vi "STED Control V9.vi"() -> ()   [LabVIEW 2014]
uses:
  Type Defs/Image Acquisition Parameters.ctl
  Laser Controls.ctl
  Detectors.ctl
  Type Defs/P541.ctl
  Type Defs/M227.ctl
  Type Defs/P612.ctl
  Type Defs/M686.ctl
  Type Defs/P841.ctl
  Type Defs/ASI.ctl
  Type Defs/N664_V2.ctl
  Type Defs/STED Graph Controls.ctl
  Type Defs/Display Controls.ctl
  FPGA-7842R-Reference.ctl
  Manual Controls V2.ctl
  Scan Parameters.ctl
  <vilib>/Utility/miscctls.llb/LVPositionTypeDef.ctl
  Controls/StageStates.ctl
  <vilib>/Utility/miscctls.llb/LVRectTypeDef.ctl
  <vilib>/event_ctls.llb/lveventtype.ctl
  <vilib>/Utility/file.llb/Read From Spreadsheet File (DBL).vi
  <vilib>/Utility/file.llb/Write To Spreadsheet File (DBL).vi
panel:
  in  "Laser Controls 2":T1={"Laser On Time (Ticks)"=15, "Laser Delay (Ticks)"=4}
  out "Channel 6":sgl[][](graph)
  out "Channel 5":sgl[][](graph)
  out "Channel 4":sgl[][](graph)
  out "Channel 3":sgl[][](graph)
  out "Channel 2":sgl[][](graph)
  out "Channel 1":sgl[][](graph)
  in  "Display Controls":T2
  in  "Graph Tools":T3={"Zoom Out"=FALSE, "Zoom In"=FALSE, "Reset Zoom"=FALSE, "Pan Tool"=FALSE, "Show Cursor"=FALSE, "Load File"=FALSE, "Fit Tool"=FALSE, "Smooth Tool"=FALSE, "Merge Tool"=FALSE, "Auto Scale"=FALSE, "Apply Color"=FALSE, "Color Map"=enum."Fire"}
  in  "Shutters":T4
  in  "Upper Objective Z - N664":T5={"Up N664"=FALSE, "Down N664"=FALSE, "Step Size (um)"=0.001, "Position (mm)"=0.0, "Home"=FALSE, "Save"=FALSE} {"Step Size (um)" min=0.001}
  in  "Cavity Translation Z - ASI":T6={"Up ASI"=FALSE, "Down ASI"=FALSE, "Step Size (um)"=0.001, "Z (um)"=0.001, "F (um)"=0.001, "Velocity"=0.001} caption="ASI" {"Velocity" min=0.001; "F (um)" min=0.001; "Z (um)" min=-1500.0 max=1500.0; "Step Size (um)" min=0.001}
  in  "Phase Comp Mirror - P841":T7={"Position (µm)"=0.0, "Step Size (µm)"=1.0, "Up P841"=FALSE, "Down P841"=FALSE}
  in  "Sample Stage XY - M686":T8 {"Y" format="%#_4g"; "X" format="%#_4g"}
  in  "Joystick Velocity":string(combo)
  in  "Radio Buttons":enum32{"Radio Selection 1", "Radio Selection 2"}(radio)
  in  "Bottom Objective XY - P612":T9 {"Y" format="%#_4g"; "X" format="%#_4g"}
  in  "Abort AllStage":bool
  in  "Stages":T10={"M227"=TRUE, "N664"=TRUE, "P612"=TRUE, "M686"=FALSE, "P841"=TRUE, "ASI"=FALSE}
  in  "Sample Z Coarse - M227":T11
  in  "Tab Control":T12(tab)
  in  "SLM":bool
  in  "DM":bool
  in  "Timing":bool
  in  "Camera":bool
  in  "Alignment":bool
  in  "Sample Z - P541":T13={"Step Up"=FALSE, "Step Down"=FALSE, "Z Position"=0.0, "Step Size (um)"=1.0, "Home"=FALSE, "Save"=FALSE}
  in  "Detectors":T14={"PMT"=TRUE, "Far Red (685/40 nm)"=FALSE, "Orange (624/40 nm)"=FALSE, "Green (525/50 nm)"=FALSE, "Sum All"=FALSE}
  in  "Laser Controls":T15 {"STED Power (V)" scale=0.0..10.0}
  in  "Save File Path":path=path "C:/isoSTED_Data/Temp/Test_0000.dbl"
  in  "Capture":bool
  in  "Image Acquisition Parameters":T16={"Scan Type"=enum."Beam Scanning", "Scan Mode"=enum."XY", "Fast Axis Frequency (Hz)"=15780.0, "Image Format"=256, "Line Accumulations"=100, "Frames Per Capture"=1, "Frames Accumulations"=1, "Image Dimension (um)"=[15.0, 15.0], "Number of Z Steps"=1, "Z Steps Size (um)"=1.0, "Pixel Size (nm)"=[58.59375, 58.59375]} {"Z Steps Size (um)" min=0.0; "Number of Z Steps" min=1; "Frames Accumulations" min=1; "Frames Per Capture" min=1; "Line Accumulations" min=1; "Image Format" items=["64 x 64"=64, "128 x 128"=128, "256 x 256"=256, "512 x 512"=512, "1024 x 1024"=1024, "2048 x 2048"=2048]}
  in  "Live":bool
  in  "Exit":bool
  # "Sample Stage XY - M686 (0~25 mm)"
  # "XY"
  # "Z"
  # "Length"
  # "Height"
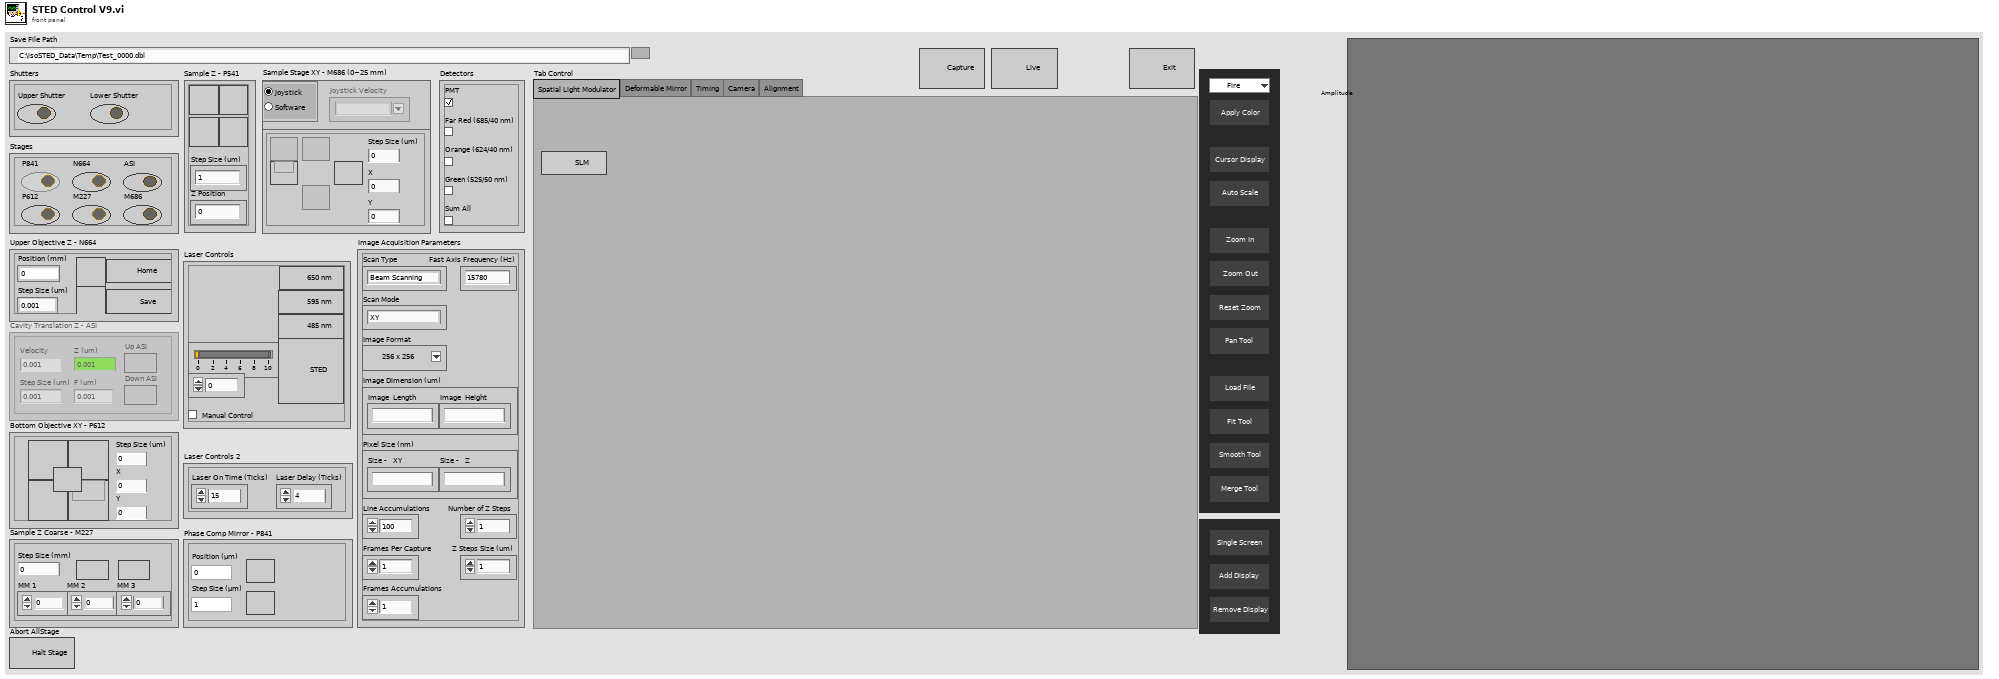
[diagram p1: front panel]
types:
  T1 = cluster{"Laser On Time (Ticks)":i8, "Laser Delay (Ticks)":i8}
  T2 = typedef "Display Controls.ctl" = cluster{"Remove Display":bool, "Add Display":bool, "Single Screen":bool}
  T3 = typedef "STED Graph Controls.ctl" = cluster{"Zoom Out":bool, "Zoom In":bool, "Reset Zoom":bool, "Pan Tool":bool, "Show Cursor":bool, "Load File":bool, "Fit Tool":bool, "Smooth Tool":bool, "Merge Tool":bool, "Auto Scale":bool, "Apply Color":bool, "Color Map":enum16{"System", "Fire", "Gray", "Red", "Green", "Blue", "Cyan", "Magenta", "Yellow", "Red-White", "Green-White", "Blue-White", "Glow"}}
  T4 = cluster{"Upper Shutter":bool, "Lower Shutter":bool}
  T5 = typedef "N664_V2.ctl" = cluster{"Up N664":bool, "Down N664":bool, "Step Size (um)":dbl, "Position (mm)":dbl, "Home":bool, "Save":bool}
  T6 = typedef "ASI.ctl" = cluster{"Up ASI":bool, "Down ASI":bool, "Step Size (um)":dbl, "Z (um)":dbl, "F (um)":dbl, "Velocity":dbl}
  T7 = typedef "P841.ctl" = cluster{"Position (µm)":dbl, "Step Size (µm)":dbl, "Up P841":bool, "Down P841":bool}
  T8 = typedef "M686.ctl" = cluster{"Home Button":bool, "Up Button":bool, "Left Button":bool, "Down Button":bool, "Right Button":bool, "Step Size (um)":dbl, "X":dbl, "Y":dbl}
  T9 = typedef "P612.ctl" = cluster{"Home Button":bool, "Up Button":bool, "Left Button":bool, "Down Button":bool, "Right Button":bool, "Step Size (um)":dbl, "X":dbl, "Y":dbl}
  T10 = cluster{"M227":bool, "N664":bool, "P612":bool, "M686":bool, "P841":bool, "ASI":bool}
  T11 = typedef "M227.ctl" = cluster{"Up M227":bool, "Down M227":bool, "Step Size (mm)":dbl, "MM 1":dbl, "MM 2":dbl, "MM 3":dbl}
  T12 = enum32{"Spatial Light Modulator", "Deformable Mirror", "Timing", "Camera", "Alignment"}
  T13 = typedef "P541.ctl" = cluster{"Step Up":bool, "Step Down":bool, "Z Position":dbl, "Step Size (um)":dbl, "Home":bool, "Save":bool}
  T14 = typedef "Detectors.ctl" = cluster{"PMT":bool, "Far Red (685/40 nm)":bool, "Orange (624/40 nm)":bool, "Green (525/50 nm)":bool, "Sum All":bool}
  T15 = typedef "Laser Controls.ctl" = cluster{"STED Power (V)":dbl, "STED":bool, "650 nm":bool, "590 nm":bool, "485 nm":bool, "Manual Control":bool}
  T16 = typedef "Image Acquisition Parameters.ctl" = cluster{"Scan Type":enum16{"Sample Scanning", "Beam Scanning"}, "Scan Mode":enum16{"XY", "XZ", "YZ", "XYZ"}, "Fast Axis Frequency (Hz)":dbl, "Image Format":u16, "Line Accumulations":u16, "Frames Per Capture":u16, "Frames Accumulations":u16, "Image Dimension (um)":dbl[], "Number of Z Steps":u8, "Z Steps Size (um)":dbl, "Pixel Size (nm)":dbl[]}
  T17 = typedef "Scan Parameters.ctl" = cluster{"Fast_Ax_Amp_V":dbl, "Fast_Ax_Off_V":dbl, "Slow_Ax_Amp_V":dbl, "Slow_Ax_Off_V ":dbl, "Slow_Ax_Max_V_VperS":dbl, "Slow_Ax1_Del25ns":i32, "Slow_Ax2_Del25ns":i32, "Stage_X_Off_V":dbl, "Stage_Y_Off_V":dbl, "Stage_Z_Off_V":dbl, "Galvo1_Off_V":dbl, "Galvo2_Off_V":dbl, "Last_Scan_Mode":enum16{"XY", "XZ", "YZ", "XYZ"}, "Current_Scan_Mode":enum16{"XY", "XZ", "YZ", "XYZ"}, "Fly_Back_Lines":u16, "Linear_Ramp_End":u32, "Z_Step_I16":i16, "Z_Start_I16":i16, "Laser_States _U32":u32, "590_Voltage_I16":i16, "775_AOM_Volt_I16":i16, "Blanking OFF":bool, "Unused_Axis_I16":i16}
  T18 = typedef "Manual Controls V2.ctl" = cluster{"Galvo 1 Position (I16)":i16, "Galvo 2 Position (I16)":i16, "X Axis Voltage (I16)":i16, "Y Axis Voltage (I16)":i16, "Z Axis Voltage (I16)":i16, "Res Mirror Amp (I16)":i16, "Res Mirror Mute":bool, "Upper Shutter":bool, "Lower Shutter":bool}
  T19 = typedef "FPGA-7842R-Reference.ctl" = enum16{"Stage Control", "Laser Control", "Unused Axis I16", "Exit", "Set Res Mirror", "Set Galvo", "Default", "Close FPGA", "Stop Waveforms", "Start Waveforms", "Shutter Control", "Initialize"}
  T20 = enum8{"Enabled", "Disabled", "Disabled and Grayed Out"}
  T21 = typedef "StageStates.ctl" = enum16{"POSITION", "MVR", "MOVE", "HALT", "ONTARGET", "ERROR", "EXIT", "HOME", "ZEROPOS", "NANOPOS", "QUIT", "ANALOG"}
  T22 = typedef "LVRectTypeDef.ctl" = cluster{"Left":i16, "Top":i16, "Right":i16, "Bottom":i16}
  T23 = enum32{"Invalid", "Standard", "Closed", "Hidden", "Minimized", "Maximized"}
  T24 = typedef "lveventtype.ctl" = enum32{"Null", "Timeout", "Annotation Menu Selection", "Annotation Menu Selection?", "App Instance Close", "App Instance Close?", "Autoscale Range Change", "Bookmark Info Change", "Cell Edit", "Cell Edit?", "Cursor Grab", "Cursor Grab?", "Cursor Menu Selection", "Cursor Menu Selection?", "Cursor Move", "Cursor Release", "Data Change", "Direction Change", "Display State Change", "Drag Ended", "Drag Enter", "Drag Leave", "Drag Over", "Drag Source Update", "Drag Starting", "Drag Starting?", "Drop", "Exec State Change", "Key Down", "Key Down?", "Key Repeat", "Key Repeat?", "Key Up", "Listbox Double Click", "Menu Activation?", "Menu Selection (App)", "Menu Selection? (App)", "Menu Selection (User)", "Mouse Down", "Mouse Down?", "Mouse Enter", "Mouse Leave", "Mouse Move", "Mouse Up", "Mouse Wheel", "NI Security User Change (App)", "Pane Size", "Panel Close", "Panel Close?", "Panel Resize", "Plot Attribute Change", "Scale Range Change", "Shortcut Menu Activation?", "Shortcut Menu Selection (App)", "Shortcut Menu Selection? (App)", "Shortcut Menu Selection (User)", "Tree Double Click", "Tree Drag", "Tree Drag?", "Tree Drop", "Tree Drop?", "Tree Item Close", "Tree Item Close?", "Tree Item Open", "Tree Item Open?", "User Event", "Value Change"}
  T25 = typedef "LVPositionTypeDef.ctl" = cluster{"Left":i32, "Top":i32}
  T26 = cluster{"Upper Shutter":bool, "Upper Shutter":bool}
  T27 = cluster{bool, bool, dbl, "Numeric":dbl, "Numeric":dbl, "Numeric":dbl}
  T28 = cluster{"Down_N664":bool, "Down_N664":bool, "Step Size (um)":dbl, "Numeric":dbl, bool, bool}
  T29 = cluster{bool, bool, bool, bool, bool, dbl, "Numeric":dbl, "Numeric":dbl}
  T30 = cluster{"Scan Type":bool, "Scan Mode":bool, "Fast Axis Frequency (Hz)":bool, "Image Format":bool, "Line Accumulations":bool, "Frames Per Capture":bool, "Frames Accumulations":bool, "Image Dimension (um)":bool[], "Number of Z Steps":bool, "Z Steps Size (um)":bool, "Pixel Size (nm)":bool[]}
  T31 = typedef "LVAllMonitorsDisplayTypeDef.ctl" = cluster{"Bounds":cluster{"Left":i16, "Top":i16, "Right":i16, "Bottom":i16}, "Depth":i16}[]
  T32 = cluster{"Bounds":cluster{"Left":i16, "Top":i16, "Right":i16, "Bottom":i16}, "Depth":i16}
  T33 = enum16{"System", "Fire", "Gray", "Red", "Green", "Blue", "Cyan", "Magenta", "Yellow", "Red-White", "Green-White", "Blue-White", "Glow"}
  T34 = typedef "LVPointDoubleTypeDef.ctl" = cluster{"Cursor X":dbl, "Cursor Y":dbl}
  T35 = typedef "LVRangeTypeDef.ctl" = cluster{"Minimum":dbl, "Maximum":dbl, "Increment":dbl, "Minor Increment":dbl, "Start":dbl}
  T36 = typedef "IMAQ Image.ctl" = refnum<image>
  T37 = typedef "Waveform Data.ctl" = cluster{"Waveform Scan Parameters":cluster{"Scanning Mode":u8, "Fast Axis WF Length (Elements)":i32, "Fast Axis Sample Period (Ticks)":u32, "Slow Axis 1 WF Length (Elements)":i32, "Slow Axis 1 Sample Period (Ticks)":u32, "Slow Axis 1 Delay (25 ns) Steps":i32, "Slow Axis 2 WFLength (Elements)":i32, "Slow Axis 2 Sample Period (Ticks)":u32, "Slow Axis 2 Delay (25 ns) Steps":i32}, "Fast Axis Waveform":dbl[], "Slow Axis 1 Waveform":dbl[], "Slow Axis 2 Waveform":dbl[]}
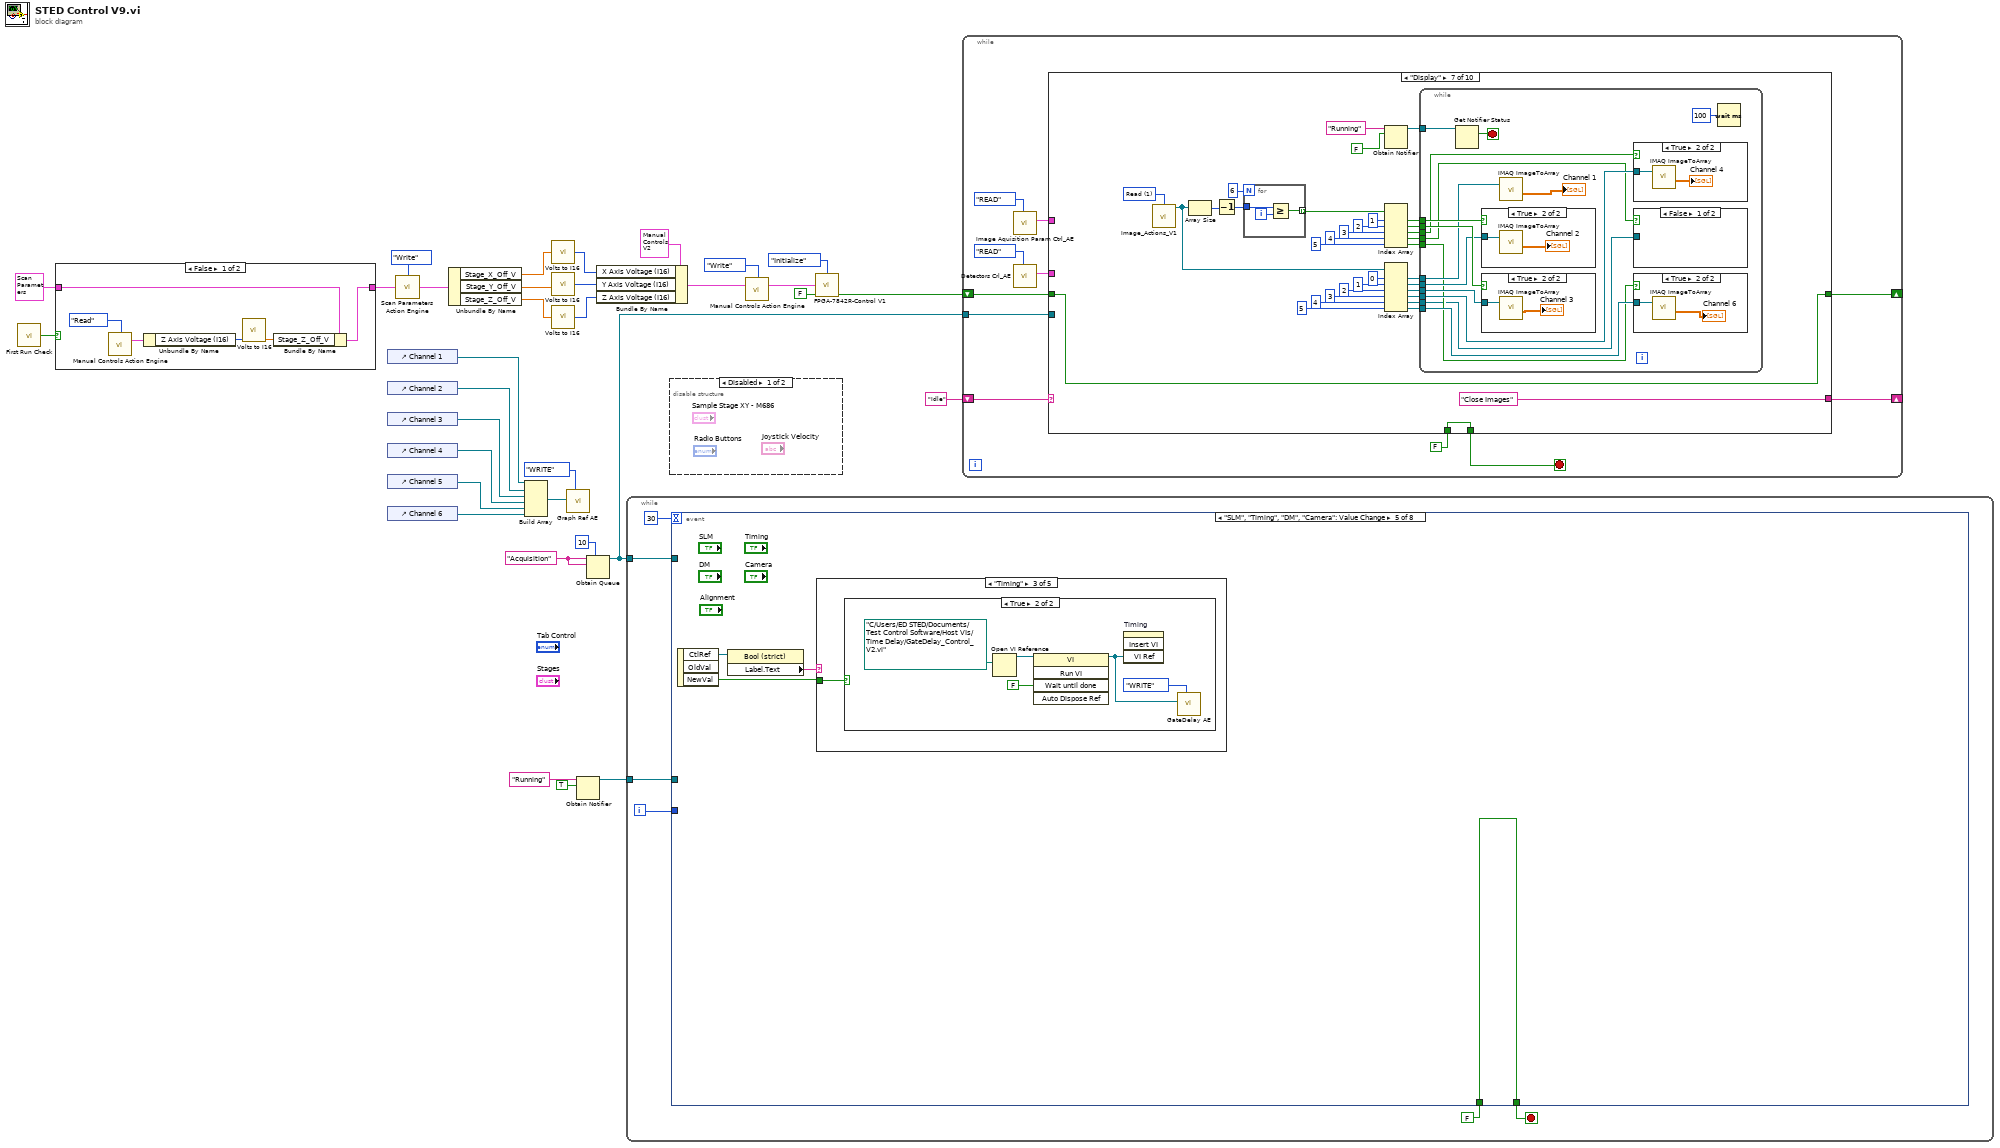
[diagram p0: block diagram]
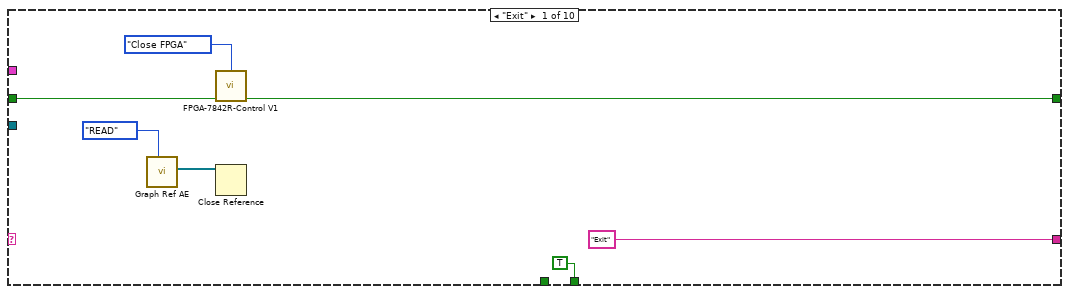
[diagram p4: hidden frame]
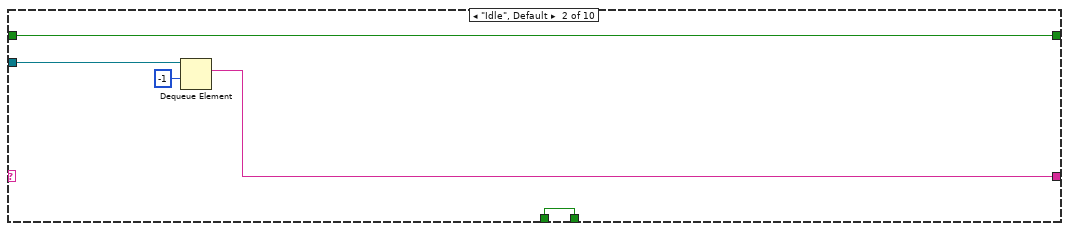
[diagram p5: hidden frame]
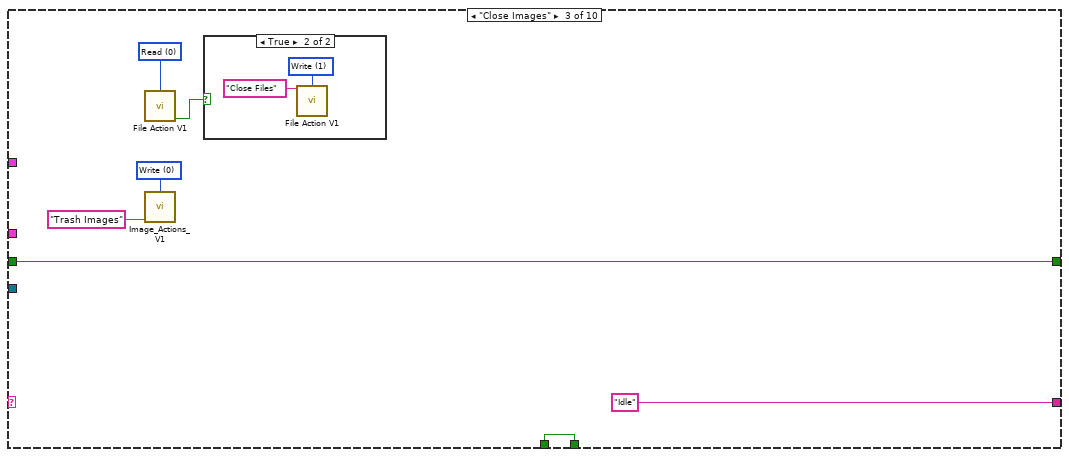
[diagram p6: hidden frame]
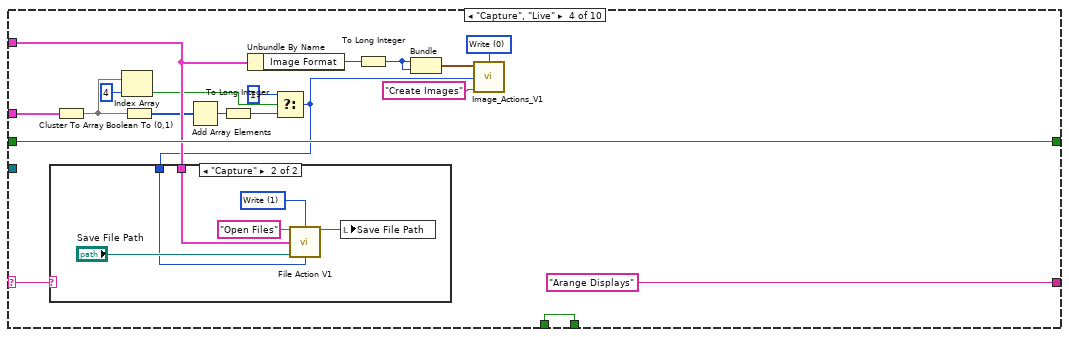
[diagram p8: hidden frame]
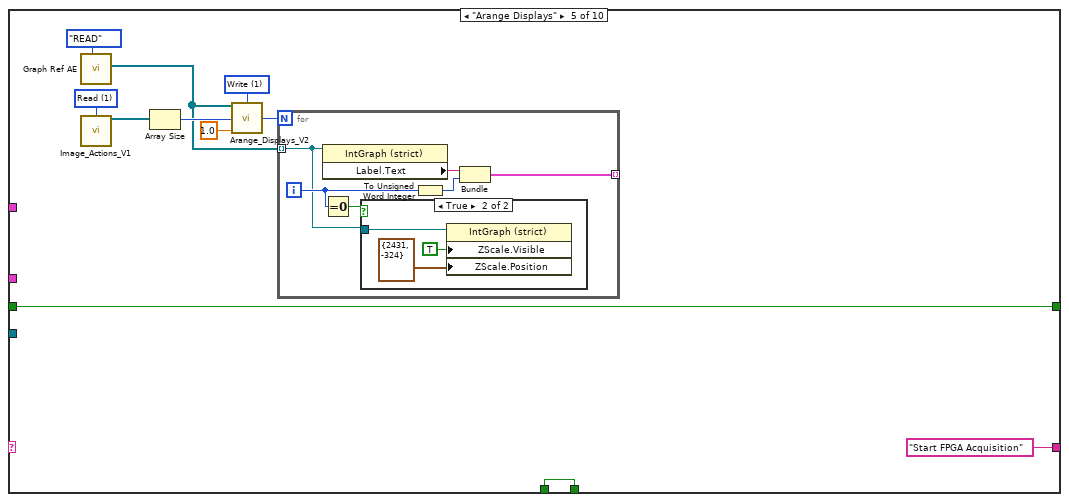
[diagram p10: hidden frame]
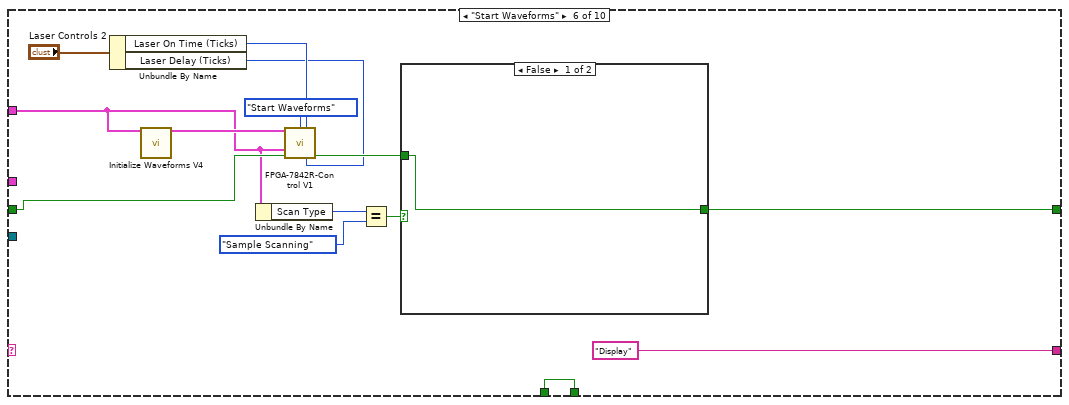
[diagram p12: hidden frame]
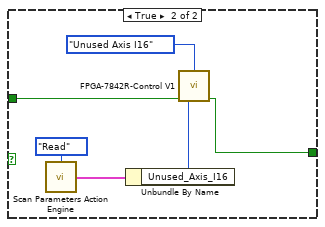
[diagram p13: hidden frame]
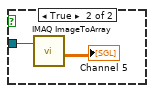
[diagram p15: hidden frame]
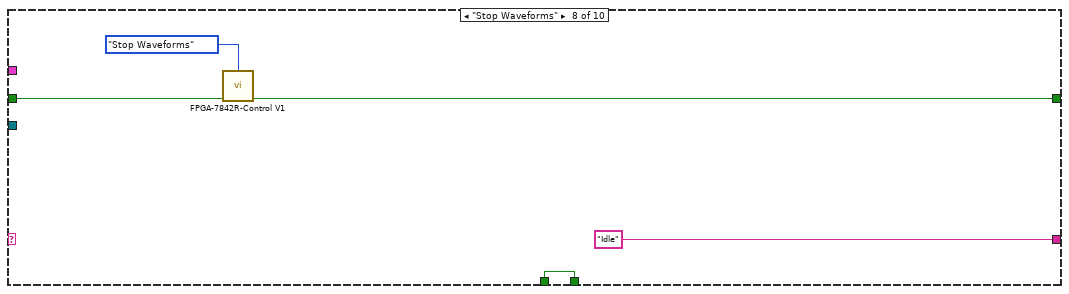
[diagram p19: hidden frame]
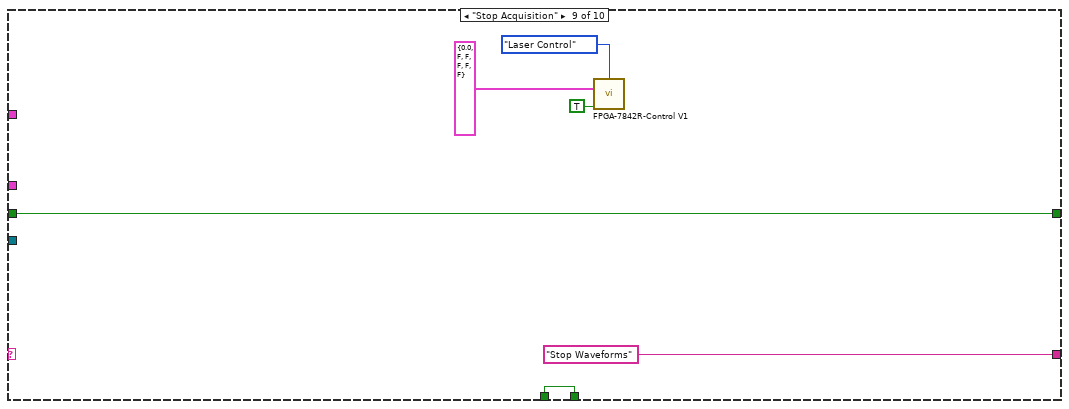
[diagram p20: hidden frame]
diagram:
  w16 = "Acquisition" ("name (unnamed)")
  n1 = call "First Run Check.vi"() -> ("First Run?"=w10:bool)  [unwired: 15 in]
  n2 = case shown="False" w10 {
    tunnel: T17 {"Fast_Ax_Amp_V"=0.0, "Fast_Ax_Off_V"=0.0, "Slow_Ax_Amp_V"=0.0, "Slow_Ax_Off_V "=0.0, "Slow_Ax_Max_V_VperS"=0.0, "Slow_Ax1_Del25ns"=0, "Slow_Ax2_Del25ns"=0, "Stage_X_Off_V"=5.0, "Stage_Y_Off_V"=5.0, "Stage_Z_Off_V"=5.0, "Galvo1_Off_V"=0.0, "Galvo2_Off_V"=0.0, "Last_Scan_Mode"=enum."XY", "Current_Scan_Mode"=enum."XY", "Fly_Back_Lines"=0, "Linear_Ramp_End"=0, "Z_Step_I16"=0, "Z_Start_I16"=0, "Laser_States _U32"=0, "590_Voltage_I16"=0, "775_AOM_Volt_I16"=0, "Blanking OFF"=FALSE, "Unused_Axis_I16"=16384} ("Scan Parameters IN") -> [w39 w40]
    tunnel: [w34 w40] -> w8
    frame False {
      n3 = call "Manual Controls Action Engine.vi"("Action"=enum16{"Read", "Write"}."Read") -> ("Manual Controls Out"=w37:T18)  [unwired: 14 in]
      n4 = Unbundle By Name(w37) -> ("Z Axis Voltage (I16)"=w38:i16)
      n5 = call "Volts to I16.vi"("Volatge (I16)"=w38) -> ("Voltage (V)"=w35:dbl)  [unwired: 13 in, 1 out]
      n6 = Bundle By Name(cluster=w39, "Stage_Z_Off_V"=w35) -> (w34:T17)
    }
    frame True {
    }
  }
  n7 = control-ref of="Channel 1"() -> (w5:refnum<vi>)
  n8 = control-ref of="Channel 2"() -> (w6:refnum<vi>)
  n9 = control-ref of="Channel 3"() -> (w7:refnum<vi>)
  n10 = control-ref of="Channel 4"() -> (w2:refnum<vi>)
  n11 = control-ref of="Channel 5"() -> (w4:refnum<vi>)
  n12 = control-ref of="Channel 6"() -> (w3:refnum<vi>)
  n13 = call "Scan Parameters Action Engine.vi"("Action"=enum16{"Read", "Write"}."Write", "Scan Parameters IN"=w8) -> ("Scan Parameters OUT"=w26:T17)  [unwired: 13 in]
  n14 = Unbundle By Name(w26) -> ("Stage_X_Off_V"=w22:dbl, "Stage_Y_Off_V"=w21:dbl, "Stage_Z_Off_V"=w20:dbl)
  n15 = Build Array(w5, w6, w7, w2, w4, w3) -> (w1:refnum<vi>[])
  n16 = call "Volts to I16.vi"("Voltage (V)"=w22) -> ("I16"=w23:i16)  [unwired: 13 in, 1 out]
  n17 = call "Volts to I16.vi"("Voltage (V)"=w21) -> ("I16"=w24:i16)  [unwired: 13 in, 1 out]
  n18 = call "Volts to I16.vi"("Voltage (V)"=w20) -> ("I16"=w25:i16)  [unwired: 13 in, 1 out]
  n19 = call "Graph Ref AE.vi"("Action"=enum16{"READ", "WRITE"}."WRITE", "Graph Ref In"=w1) -> ()  [unwired: 9 in, 1 out]
  n20 = Obtain Notifier(name (unnamed)="Running", notification data type=TRUE) -> (notifier out=w12:refnum<notifier>)  [unwired: 2 in, 2 out]
  n21 = Obtain Queue(max queue size (-1, unlimited)=10, name (unnamed)=w16, element data type=w16) -> (queue out=w18:refnum<queue>)  [unwired: 2 in, 2 out]
  n22 = Bundle By Name(cluster=T18 {"Galvo 1 Position (I16)"=-280, "Galvo 2 Position (I16)"=0, "X Axis Voltage (I16)"=16384, "Y Axis Voltage (I16)"=16384, "Z Axis Voltage (I16)"=16384, "Res Mirror Amp (I16)"=0, "Res Mirror Mute"=FALSE, "Upper Shutter"=FALSE, "Lower Shutter"=FALSE} ("Manual Controls"), "X Axis Voltage (I16)"=w23, "Y Axis Voltage (I16)"=w24, "Z Axis Voltage (I16)"=w25) -> (w27:T18)
  n23 = while {
    tunnel: w18 -> [w44]
    tunnel: w12 -> [w41]
    i -> [w42]
    stop <- w46 stop-if-true
    n24 = event shown="[4] \"SLM\", \"Timing\", \"DM\", \"Camera\": Value Change" {
      selector: _ -> [_ _ _ _ _ _ _ _]
      dyn-events: _ -> [_ _ _ _ _ _ _ _]
      timeout: 30 -> [_ _ _ _ _ _ _ _]
      tunnel: [w54 w183 w196 w322 w601 w678 w872 w925] -> w46
      tunnel: FALSE -> [w54 w183 w196 w322 w601 w678 w872 _]
      tunnel: w44 -> [w51 w182 _ _ _ _ _ w924]
      tunnel: w42 -> [w49 _ _ _ _ _ _ _]
      tunnel: w41 -> [w47 w175 _ _ _ _ _ w918]
      event Timeout {
        n25 = event-data() -> ()  [unwired: 1 in, 3 out]
        n26 = Equal To 0?(x=w49) -> (x = 0?=w48:bool)
        n27 = Get Notifier Status(notifier=w47) -> (current notification=w53:bool)  [unwired: 1 in, 4 out]
        n28 = case shown="True" w48 {
          frame False {
            w55 = enum16{"WRITE", "READ", "HOME", "SAVE HOME"}."READ" ("Enum")
            n29 = call "Image Aquisition Param Ctrl_AE.vi"("Action"=enum16{"READ", "WRITE"}."READ") -> ("Image Acquisition Parameters Out"=w83:T16)  [unwired: 10 in]
            n30 = call "Detectors Crl_AE.vi"("Action"=enum16{"READ", "WRITE"}."READ") -> ("Detectors Parameters Out"=w84:T14)  [unwired: 10 in]
            n31 = call "LASERs_ Crl_AE.vi"("Action"=enum16{"READ", "WRITE"}."READ") -> ("Detectors Parameters Out"=w85:T15)  [unwired: 10 in]
            n32 = local write "Image Acquisition Parameters"(w83) -> ()
            n33 = local write "Detectors"(w84) -> ()
            n34 = local write "Laser Controls"(w85) -> ()
            n35 = call "Stage_position_ae.vi"("StageID"="M227", "Enum"=w55) -> ("Position Out"=w61:dbl[])  [unwired: 8 in, 1 out]
            n36 = call "Stage_position_ae.vi"("StageID"="P612", "Enum"=w55) -> ("Position Out"=w78:dbl[])  [unwired: 8 in, 1 out]
            n37 = call "Stage_position_ae.vi"("StageID"="P841", "Enum"=w55) -> ("Position Out"=w71:dbl[])  [unwired: 8 in, 1 out]
            n38 = call "Stage_position_ae.vi"("StageID"="N664", "Enum"=w55) -> ("Position Out"=w65:dbl[])  [unwired: 8 in, 1 out]
            n39 = Index Array(array=w65, index=0) -> (element=w64:dbl)
            n40 = Index Array(array=w71, index=0) -> (element=w68:dbl)
            n41 = Index Array(array=w78, index #1=0 ("index"), index #2=1 ("index"), index #3=2 ("index")) -> (element #1=w77:dbl, element #2=w74:dbl, element #3=w72:dbl)
            n42 = Index Array(array=w61, index #1=0 ("index"), index #2=1 ("index"), index #3=2 ("index")) -> (element #1=w58:dbl, element #2=w57:dbl, element #3=w56:dbl)
            n43 = property on="Position (µm)" class="DigNum (strict)"("Value"=w68) -> ()  [unwired: 2 in, 2 out]
            n44 = property on="Position (mm)" class="DigNum (strict)"("Value"=w64) -> ()  [unwired: 2 in, 2 out]
            n45 = property on="X" class="DigNum (strict)"("Value"=w77) -> ()  [unwired: 2 in, 2 out]
            n46 = property on="Y" class="DigNum (strict)"("Value"=w74) -> ()  [unwired: 2 in, 2 out]
            n47 = property on="MM 1" class="DigNum (strict)"("Value"=w58) -> ()  [unwired: 2 in, 2 out]
            n48 = property on="MM 2" class="DigNum (strict)"("Value"=w57) -> ()  [unwired: 2 in, 2 out]
            n49 = property on="Z Position" class="DigNum (strict)"("Value"=w72) -> ()  [unwired: 2 in, 2 out]
            n50 = property on="MM 3" class="DigNum (strict)"("Value"=w56) -> ()  [unwired: 2 in, 2 out]
          }
          frame True {
            w87 = enum16{"WRITE", "READ", "HOME", "SAVE HOME"}."SAVE HOME" ("Enum")
            w99 = FALSE ("Upper Shutter")
            n51 = local read "Image Acquisition Parameters"() -> (w106:T16)
            n52 = local read "Laser Controls"() -> (w104:T15)
            n53 = local read "Detectors"() -> (w103:T14)
            n54 = Bundle("Upper Shutter"=w99, "Upper Shutter"=w99) -> (w100:T26)  [unwired: 1 in]
            n55 = property on="Shutters" class="Clust (strict)"("Value"=w100) -> ()  [unwired: 2 in, 2 out]
            n56 = call "Image Aquisition Param Ctrl_AE.vi"("Action"=enum16{"READ", "WRITE"}."WRITE", "Image Acquisition Parameters In"=w106) -> ()  [unwired: 9 in, 1 out]
            n57 = call "Detectors Crl_AE.vi"("Action"=enum16{"READ", "WRITE"}."WRITE", "Detectors Parameters In"=w103) -> ()  [unwired: 9 in, 1 out]
            n58 = call "LASERs_ Crl_AE.vi"("Action"=enum16{"READ", "WRITE"}."WRITE", "Detectors Parameters In"=w104) -> ()  [unwired: 9 in, 1 out]
            n59 = property on="Stages" class="Clust (strict)"() -> ("Controls[]"=w101:refnum<vi>[])  [unwired: 2 in, 2 out]
            n60 = for {
              tunnel: w101 -> [w111] mode=indexing
              n61 = property class="Ctl"(reference=w111) -> ("Label.Text"=w109:string, "Value"=w113:variant)  [unwired: 1 in, 2 out]
              n62 = Variant To Data(type=TRUE, Variant=w113) -> (data=w110:bool)  [unwired: 1 in, 1 out]
              n63 = call "All_Stages_Aloha.vi"("Aloha"=w110, "Stage ID"=w109) -> ("Position Out"=w108:dbl[])  [unwired: 9 in]
              n64 = case shown="\"N664\"" w109 {
                tunnel: w108 -> [_ w120 w128 w135 w145 w156 w166]
                frame "0", Default {
                }
                frame "M227" {
                  w124 = FALSE
                  n65 = Index Array(array=w120, index #1=0 ("index"), index #2=1 ("index"), index #3=2 ("index")) -> (element #1=w116:dbl, element #2=w115:dbl, element #3=w114:dbl)
                  n66 = Bundle(w124, w124, 0.0, "Numeric"=w116, "Numeric"=w115, "Numeric"=w114) -> (w122:T27)  [unwired: 1 in]
                  n67 = To Variant(anything=w122) -> (Variant=w121:variant)
                  n68 = property on="Sample Z Coarse - M227" class="Clust"("Value"=w121) -> ()  [unwired: 2 in, 2 out]
                }
                frame "N664" {
                  w125 = FALSE
                  w131 = FALSE ("Down_N664")
                  n69 = Index Array(array=w128, index=0) -> (element=w129:dbl)
                  n70 = Bundle("Down_N664"=w131, "Down_N664"=w131, "Step Size (um)"=1.0, "Numeric"=w129, w125, w125) -> (w127:T28)  [unwired: 1 in]
                  n71 = To Variant(anything=w127) -> (Variant=w126:variant)
                  n72 = property on="Upper Objective Z - N664" class="Clust"("Value"=w126) -> ()  [unwired: 2 in, 2 out]
                }
                frame "P612" {
                  w143 = FALSE
                  n73 = Index Array(array=w135, index #1=0, index #2=1, index #3=2 ("index")) -> (element #1=w140:dbl, element #2=w138:dbl, element #3=w133:dbl)
                  n74 = Bundle(w143, w143, w143, w143, w143, 1.0, "Numeric"=w140, "Numeric"=w138) -> (w139:T29)  [unwired: 1 in]
                  n75 = To Variant(anything=w139) -> (Variant=w134:variant)
                  n76 = property on="Bottom Objective XY - P612" class="Clust"("Value"=w134) -> ()  [unwired: 2 in, 2 out]
                  n77 = property on="Z Position" class="DigNum (strict)"("Value"=w133) -> ()  [unwired: 2 in, 2 out]
                }
                frame "M686" {
                  w154 = FALSE
                  n78 = Index Array(array=w145, index #1=0, index #2=1) -> (element #1=w151:dbl, element #2=w146:dbl)
                  n79 = Bundle(w154, w154, w154, w154, w154, 10.0, "Numeric"=w151, "Numeric"=w146) -> (w150:T29)  [unwired: 1 in]
                  n80 = To Variant(anything=w150) -> (Variant=w144:variant)
                  n81 = property on="Joystick Velocity" class="CmbBox"("DisabledEnum"=T20."Disabled and Grayed Out" ("Disabled")) -> ()  [unwired: 2 in, 2 out]
                  n82 = property on="Radio Buttons" class="RadioBtnsControl (strict)"("Value"=enum32{"Radio Selection 1", "Radio Selection 2"}."Radio Selection 2" ("Radio Buttons")) -> ()  [unwired: 2 in, 2 out]
                  n83 = property on="Sample Stage XY - M686" class="Clust"("Value"=w144) -> ()  [unwired: 2 in, 2 out]
                }
                frame "P841" {
                  n84 = Index Array(array=w156, index=0) -> (element=w155:dbl)
                  n85 = property on="Position (µm)" class="DigNum (strict)"("Value"=w155) -> ()  [unwired: 2 in, 2 out]
                }
                frame "ASI" {
                  w162 = FALSE
                  n86 = Add Array Elements(numeric array=w166) -> (sum=w168:dbl)
                  n87 = Index Array(array=w166, index #1=0 ("index"), index #2=1 ("index")) -> (element #1=w161:dbl, element #2=w160:dbl)
                  n88 = Divide(x=w168, y=2000.0) -> ()  [unwired: 1 out]
                  n89 = Bundle By Name(cluster=T6 {"Up ASI"=FALSE, "Down ASI"=FALSE, "Step Size (um)"=0.001, "Z (um)"=0.001, "F (um)"=0.001, "Velocity"=0.001} ("Cavity Translation Z - ASI"), "Up ASI"=w162, "Down ASI"=w162, "Step Size (um)"=1.0, "Z (um)"=w161, "F (um)"=w160, "Velocity"=0.1) -> (w158:T6)
                  n90 = To Variant(anything=w158) -> (Variant=w159:variant)
                  n91 = property on="Cavity Translation Z - ASI" class="Clust"("Value"=w159) -> ()  [unwired: 2 in, 2 out]
                }
              }
            }
            n92 = call-poly <vilib>:"Read From Spreadsheet File.vi"("format (%.3f)"="%.4f", "number of rows (all:-1)"=1, "file path (dialog if empty)"=path "C:/Users/ED STED/Documents/Test Control Software/Host VIs/Stages/Stage Positions/home position.csv") -> ("first row"=w96:dbl[])  [unwired: 4 in, 4 out]
            n93 = Index Array(array=w96, index #1=0 ("index"), index #2=1 ("index")) -> (element #1=w92:dbl, element #2=w93:dbl)
            n94 = Build Array(w92) -> (w91:dbl[])
            n95 = Build Array(w93) -> (w89:dbl[])
            n96 = call "Stage_position_ae.vi"("Position In"=w91, "StageID"="P541", "Enum"=w87) -> ()  [unwired: 7 in, 2 out]
            n97 = call "Stage_position_ae.vi"("Position In"=w89, "StageID"="N664", "Enum"=w87) -> ()  [unwired: 7 in, 2 out]
          }
        }
        n98 = local read "Capture"() -> (w52:bool)
        n99 = And(x=w53, y=w52) -> (x .and. y?=w50:bool)
        n100 = case shown="False" w50 {
          tunnel: w51 -> [_ w173]
          frame False {
          }
          frame True {
            n101 = local write "Capture"(FALSE ("Capture")) -> ()
            n102 = Enqueue Element(queue=w173, element="Stop Acquisition" ("f")) -> ()  [unwired: 2 in, 3 out]
            n103 = property on="Live" class="Bool (strict)"("DisabledEnum"=T20."Enabled" ("Disabled")) -> ()  [unwired: 2 in, 2 out]
          }
        }
      }
      event "Live", "Capture": Value Change {
        n104 = event-data() -> ("CtlRef"=w181:refnum<vi>, "NewVal"=w176:bool)  [unwired: 1 in]
        n105 = Not(x=w176) -> (.not. x?=w179:bool)
        n106 = property class="Bool (strict)"(reference=w181) -> ("Label.Text"=w177:string)  [unwired: 1 in, 2 out]
        n107 = Send Notification(notification=w179, notifier=w175) -> ()  [unwired: 1 in, 2 out]
        n108 = case shown="\"Live\"" w177 {
          tunnel: w176 -> [_ w185 w189]
          frame "False", Default {
          }
          frame "Live" {
            n109 = case shown="True" w185 {
              tunnel: [T20."Enabled" ("Disabled") T20."Disabled and Grayed Out" ("Disabled")] -> w184
              frame False {
              }
              frame True {
              }
            }
            n110 = property on="Capture" class="Bool (strict)"("DisabledEnum"=w184) -> ()  [unwired: 2 in, 2 out]
            n111 = property on="Exit" class="Bool"("DisabledEnum"=w184) -> ()  [unwired: 2 in, 2 out]
          }
          frame "Capture" {
            n112 = case shown="True" w189 {
              tunnel: [T20."Enabled" ("Disabled") T20."Disabled and Grayed Out" ("Disabled")] -> w188
              frame False {
              }
              frame True {
              }
            }
            n113 = property on="Live" class="Bool (strict)"("DisabledEnum"=w188) -> ()  [unwired: 2 in, 2 out]
            n114 = property on="Exit" class="Bool"("DisabledEnum"=w188) -> ()  [unwired: 2 in, 2 out]
          }
        }
        n115 = Select(t=w177, s=w176, f="Stop Acquisition") -> (s? t:f=w178:string)
        n116 = Enqueue Element(queue=w182, element=w178) -> ()  [unwired: 2 in, 3 out]
      }
      event "Shutters": Value Change {
        n117 = event-data() -> ("CtlRef"=w195:refnum<vi>, "NewVal"=w194:variant, "OldVal"=w193:variant)  [unwired: 1 in]
        n118 = property class="Clust"(reference=w195) -> ("Label.Text"=w192:string)  [unwired: 1 in, 2 out]
        n119 = case shown="\"Shutters\"" w192 {
          tunnel: w194 -> [_ w207 _ _ _]
          tunnel: w193 -> [_ w205 _ _ _]
          frame Default {
          }
          frame "Image Acquisition Parameters" {
            n120 = Variant To Data(type="Image Acquisition Parameters", Variant=w207) -> (data=w204:T16)  [unwired: 1 in, 1 out]
            n121 = Variant To Data(type=w204, Variant=w205) -> (data=w203:T16)  [unwired: 1 in, 1 out]
            n122 = Not Equal?(x=w204, y=w203) -> (x != y?=w229:T30)
            n123 = Unbundle By Name(w229) -> ("Image Dimension (um)"=w214:bool[], "Image Format"=w212:bool, "Pixel Size (nm)"=w213:bool[])
            n124 = Or Array Elements(Boolean array=w214) -> (logical OR=w218:bool)
            n125 = Or Array Elements(Boolean array=w213) -> (logical OR=w217:bool)
            n126 = Build Array(w218, w212, w217) -> (w216:bool[])
            n127 = Boolean Array To Number(Boolean array=w216) -> (number=w215:u32)
            n128 = case shown="1, 2" w215 {
              tunnel: w214 -> [_ w251 _]
              tunnel: w204 -> [w239 w244 w259]
              tunnel: [w239 w242 w257] -> w211
              tunnel: w213 -> [_ _ w256]
              tunnel: [w238 w241 w255] -> w210
              tunnel: [w237 w240 w254] -> w208
              frame 0, Default {
                n129 = Unbundle By Name(w239) -> ("Image Dimension (um)"=w238:dbl[], "Scan Mode"=w237:enum16{"XY", "XZ", "YZ", "XYZ"})
              }
              frame 1, 2 {
                # "Image Dimension or Format Change"
                n130 = Unbundle By Name(w244) -> ("Image Dimension (um)"=w250:dbl[], "Image Format"=w248:u16, "Scan Mode"=w240:enum16{"XY", "XZ", "YZ", "XYZ"})
                n131 = for {
                  tunnel: w251 -> [w253] mode=indexing
                  tunnel: w250 -> [w252] mode=indexing
                  tunnel: [w252] -> w249
                  stop <- w253 stop-if-true
                }
                n132 = To Double Precision Float(number=w248) -> (double precision float=w247:dbl)
                n133 = Build Array(w249, w249) -> (w241:dbl[])
                n134 = Divide(x=w241, y=w247) -> (x/y=w246:dbl[])
                n135 = Multiply(x=w246, y=1000.0) -> (x*y=w243:dbl[])
                n136 = Bundle By Name(cluster=w244, "Image Dimension (um)"=w241, "Pixel Size (nm)"=w243) -> (w242:T16)
              }
              frame 4 {
                # "Pixel Size Change"
                n137 = Unbundle By Name(w259) -> ("Pixel Size (nm)"=w265:dbl[], "Image Format"=w263:u16, "Scan Mode"=w254:enum16{"XY", "XZ", "YZ", "XYZ"})
                n138 = for {
                  tunnel: w256 -> [w267] mode=indexing
                  tunnel: w265 -> [w266] mode=indexing
                  tunnel: [w266] -> w264
                  stop <- w267 stop-if-true
                }
                n139 = Build Array(w264, w264) -> (w258:dbl[])
                n140 = To Double Precision Float(number=w263) -> (double precision float=w262:dbl)
                n141 = Multiply(x=w258, y=w262) -> (x*y=w261:dbl[])
                n142 = Multiply(x=w261, y=0.001) -> (x*y=w255:dbl[])
                n143 = Bundle By Name(cluster=w259, "Pixel Size (nm)"=w258, "Image Dimension (um)"=w255) -> (w257:T16)
              }
            }
            n144 = Index Array(array=w210, index=0) -> (element=w234:dbl)
            n145 = Not Equal?(x=enum16{"XY", "XZ", "YZ", "XYZ"}."YZ" ("y"), y=w208) -> (x != y?=w219:bool)
            n146 = call "Res Mirror um to Volts.vi"("Image Size (um)"=w234) -> ("Voltage (V)"=w197:dbl)
            n147 = Select(t=15780.0, s=w219, f=200.0) -> (s? t:f=w222:dbl)
            n148 = In Range and Coerce(upper limit=5.0, x=w197, lower limit=0.0) -> (coerced(x)=w199:dbl)  [unwired: 1 out]
            n149 = call "Scan Parameters Action Engine.vi"("Action"=enum16{"Read", "Write"}."Read") -> ("Scan Parameters OUT"=w200:T17)  [unwired: 14 in]
            n150 = Bundle By Name(cluster=w200, "Fast_Ax_Amp_V"=w199) -> (w198:T17)
            n151 = Bundle By Name(cluster=w211, "Fast Axis Frequency (Hz)"=w222) -> (w221:T16)
            n152 = call "Volts to I16.vi"("Voltage (V)"=w199) -> ("I16"=w233:i16)  [unwired: 13 in, 1 out]
            n153 = call "Scan Parameters Action Engine.vi"("Action"=enum16{"Read", "Write"}."Write", "Scan Parameters IN"=w198) -> ()  [unwired: 13 in, 1 out]
            n154 = call "Manual Controls Action Engine.vi"("Action"=enum16{"Read", "Write"}."Read") -> ("Manual Controls Out"=w227:T18)  [unwired: 14 in]
            n155 = Bundle By Name(cluster=w227, "Res Mirror Amp (I16)"=w233, "Res Mirror Mute"=w219) -> (w225:T18)
            n156 = call "Image Aquisition Param Ctrl_AE.vi"("Action"=enum16{"READ", "WRITE"}."WRITE", "Image Acquisition Parameters In"=w221) -> ()  [unwired: 9 in, 1 out]
            n157 = call "FPGA-7842R-Control V1.vi"("Action"=FPGA-7842R-Reference."Set Res Mirror", "Manual Controls"=w225, "Initialize"=TRUE) -> ()  [unwired: 11 in, 2 out]
            n158 = call "Manual Controls Action Engine.vi"("Action"=enum16{"Read", "Write"}."Write", "Manual Controls In"=w225) -> ()  [unwired: 13 in, 1 out]
          }
          frame "Detectors" {
            n159 = call "Detectors Crl_AE.vi"("Action"=enum16{"READ", "WRITE"}."WRITE", "Detectors Parameters In"="Detectors") -> ()  [unwired: 9 in, 1 out]
          }
          frame "Laser Controls" {
            w282 = FALSE ("element")
            n160 = Unbundle By Name("Laser Controls") -> ("STED"=w288:bool, "650 nm"=w285:bool, "590 nm"=w286:bool, "485 nm"=w287:bool, "STED Power (V)"=w279:dbl, "Manual Control"=w273:bool)
            n161 = local read "Live"() -> (w274:bool)
            n162 = call "LASERs_ Crl_AE.vi"("Action"=enum16{"READ", "WRITE"}."WRITE", "Detectors Parameters In"="Laser Controls") -> ()  [unwired: 9 in, 1 out]
            n163 = Or(x=w274, y=w273) -> (x .or. y?=w272:bool)
            n164 = In Range and Coerce(upper limit=10.0, x=w279, lower limit=0.0) -> (coerced(x)=w276:dbl)  [unwired: 1 out]
            n165 = Build Array(w288, w285, w286, w287, w282, w282, w282, w282) -> (w284:bool[])
            n166 = case shown="True" w272 {
              tunnel: "Laser Controls" -> [_ w294]
              frame False {
              }
              frame True {
                n167 = call "FPGA-7842R-Control V1.vi"("Action"=FPGA-7842R-Reference."Laser Control", "Laser Controls"=w294, "Initialize"=TRUE) -> ()  [unwired: 11 in, 2 out]
              }
            }
            n168 = Boolean Array To Number(Boolean array=w284) -> (number=w283:u32)
            n169 = To Unsigned Byte Integer(number=w283) -> (unsigned 8bit integer=w281:u8)
            n170 = call "U8_To_U32.vi"("U8 IN"=w281) -> ("U32 OUT"=w280:u32)  [unwired: 13 in, 1 out]
            n171 = call "Volts to I16.vi"("Voltage (V)"=w276) -> ("I16"=w275:i16)  [unwired: 13 in, 1 out]
            n172 = call "Scan Parameters Action Engine.vi"("Action"=enum16{"Read", "Write"}."Read") -> ("Scan Parameters OUT"=w291:T17)  [unwired: 14 in]
            n173 = Bundle By Name(cluster=w291, "Laser_States _U32"=w280, "775_AOM_Volt_I16"=w275) -> (w289:T17)
            n174 = call "Scan Parameters Action Engine.vi"("Action"=enum16{"Read", "Write"}."Write", "Scan Parameters IN"=w289) -> ()  [unwired: 13 in, 1 out]
          }
          frame "Shutters" {
            n175 = Unbundle By Name("Shutters") -> ("Upper Shutter"=w306:bool, "Lower Shutter"=w305:bool)
            n176 = Not(x=w306) -> (.not. x?=w297:bool)
            n177 = Not(x=w305) -> (.not. x?=w296:bool)
            n178 = call "Manual Controls Action Engine.vi"("Action"=enum16{"Read", "Write"}."Read") -> ("Manual Controls Out"=w301:T18)  [unwired: 14 in]
            n179 = Bundle By Name(cluster=w301, "Upper Shutter"=w297, "Lower Shutter"=w296) -> (w298:T18)
            n180 = call "Manual Controls Action Engine.vi"("Action"=enum16{"Read", "Write"}."Write", "Manual Controls In"=w298) -> ()  [unwired: 13 in, 1 out]
            n181 = call "FPGA-7842R-Control V1.vi"("Action"=FPGA-7842R-Reference."Shutter Control", "Manual Controls"=w298, "Initialize"=TRUE) -> ()  [unwired: 11 in, 2 out]
          }
        }
      }
      event Value Change {
        # "For P541 - Sample Z - Converting from Step in µm to I16 is as follows. We have (Step µw)*(10 V / 100 µm)*(32768 I16 / 10 V) = (Step µm)*(32768 I16 / 100 µm) = (Step µm)*(327.68 I16/µm)"
        n182 = event-data() -> ("CtlRef"=w320:refnum<vi>, "OldVal"=w318:variant, "NewVal"=w319:variant)  [unwired: 1 in]
        n183 = local write "Abort AllStage"(FALSE ("Abort AllStage")) -> ()
        n184 = property class="Clust"(reference=w320) -> ("Label.Text"=w317:string)  [unwired: 1 in, 2 out]
        n185 = case shown="\"Upper Objective Z - N664\"" w317 {
          tunnel: w319 -> [_ w343 w384 w411 w474 w515 w544]
          tunnel: w318 -> [_ w342 w383 w410 w475 w516 w545]
          tunnel: ["" "N664" "ASI" "P612" "P612" "P841" "M227"] -> w316
          tunnel: [dbl[] [0.0] w334 w376 w399 dbl[] [0.0] w504 w537] -> w315
          tunnel: [bool[] [FALSE] w332 w370 w400 bool[] [FALSE] bool[] [TRUE] w538] -> w314
          tunnel: [enum16{"MOVE", "MVR"}."MVR" ("MOVE/MVR") w331 w373 w402 enum16{"MOVE", "MVR"}."MVR" ("MOVE/MVR") w507 w530] -> w313
          tunnel: [0.0 ("Step Size (um)") 0.5 ("Step Size (um)") w375 0.0 ("Velocity") 0.0 ("Velocity") 10000.0 ("Velocity") 0.0 ("Velocity")] -> w309
          tunnel: [StageStates."MVR" ("Action") w329 w374 w403 StageStates."POSITION" ("Action") w508 w534] -> w307
          frame Default {
          }
          frame "Upper Objective Z - N664" {
            n186 = call "N664_Ctrl_Index.vi"("OldVal"=w342, "NewVal"=w343) -> ("Control Ref OUT"=w341:refnum<vi>, "N664 Out"=w339:T5)  [unwired: 12 in]
            n187 = property class="Ctl"(reference=w341) -> ("Label.Text"=w340:string)  [unwired: 1 in, 2 out]
            n188 = Unbundle By Name(w339) -> ("Step Size (um)"=w338:dbl, "Position (mm)"=w337:dbl)
            n189 = case shown="\"Save\"" w340 {
              tunnel: w338 -> [_ w348 w351 _ _ _]
              tunnel: [0.0 ("Step Size (um)") w347 w351 w356 w358 w363] -> w335
              tunnel: w337 -> [_ _ _ w356 w358 _]
              tunnel: [enum16{"MOVE", "MVR"}."MVR" ("MOVE/MVR") enum16{"MOVE", "MVR"}."MVR" ("MOVE/MVR") enum16{"MOVE", "MVR"}."MVR" ("MOVE/MVR") enum16{"MOVE", "MVR"}."MOVE" ("MOVE/MVR") enum16{"MOVE", "MVR"}."MOVE" ("MOVE/MVR") enum16{"MOVE", "MVR"}."MOVE" ("MOVE/MVR")] -> w331
              tunnel: [StageStates."MVR" ("Action") StageStates."MVR" ("Action") StageStates."MVR" ("Action") StageStates."MOVE" ("Action") StageStates."MOVE" ("Action") StageStates."MOVE" ("Action")] -> w329
              frame Default {
              }
              frame "Up N664" {
                n190 = Negate(x=w348) -> (-x=w347:dbl)
              }
              frame "Down N664" {
              }
              frame "Position (mm)" {
              }
              frame "Save" {
                n191 = Build Array(w358) -> (w357:dbl[])
                n192 = call "Stage_position_ae.vi"("Position In"=w357, "StageID"="N664", "Enum"=enum16{"WRITE", "READ", "HOME", "SAVE HOME"}."SAVE HOME") -> ()  [unwired: 7 in, 2 out]
              }
              frame "Home" {
                n193 = call "Stage_position_ae.vi"("StageID"="N664", "Enum"=enum16{"WRITE", "READ", "HOME", "SAVE HOME"}."HOME") -> ("Position Out"=w365:dbl[])  [unwired: 8 in, 1 out]
                n194 = Index Array(array=w365, index=0) -> (element=w363:dbl)
              }
            }
            n195 = Build Array(w335) -> (w334:dbl[])
            n196 = Build Array(TRUE) -> (w332:bool[])
          }
          frame "Cavity Translation Z - ASI" {
            n197 = call "ASI_Ctrl_Index.vi"("NewVal"=w384, "OldVal"=w383) -> ("ASI out"=w380:T6, "Control Ref OUT"=w382:refnum<vi>)  [unwired: 8 in]
            n198 = property class="Ctl"(reference=w382) -> ("Label.Text"=w381:string)  [unwired: 1 in, 2 out]
            n199 = Unbundle By Name(w380) -> ("Step Size (um)"=w379:dbl, "Z (um)"=w378:dbl, "Velocity"=w375:dbl)
            n200 = case shown="\"Z (um)\"" w381 {
              tunnel: w379 -> [_ w390 w393 _]
              tunnel: w378 -> [_ _ _ w397]
              tunnel: [0.0 ("Z (um)") w390 w394 w397] -> w377
              tunnel: [StageStates."MVR" ("Action") StageStates."MVR" ("Action") StageStates."MVR" ("Action") StageStates."MOVE" ("Action")] -> w374
              tunnel: [enum16{"MOVE", "MVR"}."MVR" ("MOVE/MVR") enum16{"MOVE", "MVR"}."MVR" ("MOVE/MVR") enum16{"MOVE", "MVR"}."MVR" ("MOVE/MVR") enum16{"MOVE", "MVR"}."MOVE" ("MOVE/MVR")] -> w373
              frame Default {
              }
              frame "Up ASI" {
              }
              frame "Down ASI" {
                n201 = Negate(x=w393) -> (-x=w394:dbl)
              }
              frame "Z (um)" {
              }
            }
            n202 = Build Array(w377) -> (w376:dbl[])
            n203 = Build Array(TRUE) -> (w370:bool[])
          }
          frame "Bottom Objective XY - P612" {
            n204 = call "P612_Ctrl_Index.vi"("OldVal"=w410, "NewVal"=w411) -> ("Control out"=w409:refnum<vi>, "P612 out"=w407:T9)  [unwired: 12 in]
            n205 = property class="Ctl"(reference=w409) -> ("Label.Text"=w408:string)  [unwired: 1 in, 2 out]
            n206 = Unbundle By Name(w407) -> ("Step Size (um)"=w406:dbl, "X"=w405:dbl, "Y"=w404:dbl)
            n207 = case shown="\"Up Button\"" w408 {
              tunnel: w406 -> [_ _ w422 w429 w433 w440 _]
              tunnel: w405 -> [_ _ _ _ _ _ w447]
              tunnel: w404 -> [_ _ _ _ _ _ w446]
              tunnel: [StageStates."MVR" ("Action") StageStates."HOME" ("Action") StageStates."MVR" ("Action") StageStates."MVR" ("Action") StageStates."MVR" ("Action") StageStates."MVR" ("Action") StageStates."MOVE" ("Action")] -> w403
              tunnel: [enum16{"MOVE", "MVR"}."MVR" ("MOVE/MVR") enum16{"MOVE", "MVR"}."MVR" ("MOVE/MVR") enum16{"MOVE", "MVR"}."MVR" ("MOVE/MVR") enum16{"MOVE", "MVR"}."MVR" ("MOVE/MVR") enum16{"MOVE", "MVR"}."MVR" ("MOVE/MVR") enum16{"MOVE", "MVR"}."MVR" ("MOVE/MVR") enum16{"MOVE", "MVR"}."MOVE" ("MOVE/MVR")] -> w402
              tunnel: [bool[] [FALSE] bool[] [TRUE, TRUE] bool[] [TRUE, FALSE] bool[] [TRUE, FALSE] bool[] [FALSE, TRUE] bool[] [FALSE, TRUE] bool[] [TRUE, TRUE]] -> w400
              tunnel: [dbl[] [0.0] dbl[] [0.0, 0.0] w421 w428 w435 w442 w448] -> w399
              frame Default {
              }
              frame "Home Button" {
              }
              frame "Up Button" {
                n208 = Build Array(w422, 0.0 ("element")) -> (w421:dbl[])
              }
              frame "Down Button" {
                n209 = Negate(x=w429) -> (-x=w426:dbl)
                n210 = Build Array(w426, 0.0 ("element")) -> (w428:dbl[])
              }
              frame "Left Button" {
                n211 = Build Array(0.0 ("element"), w433) -> (w435:dbl[])
              }
              frame "Right Button" {
                n212 = Negate(x=w440) -> (-x=w439:dbl)
                n213 = Build Array(0.0 ("element"), w439) -> (w442:dbl[])
              }
              frame "X", "Y" {
                n214 = Build Array(w447, w446) -> (w448:dbl[])
              }
            }
          }
          frame "Sample Z - P541" {
            w453 = 327.68 ("y")
            n215 = call "P541_Ctrl_Index.vi"("OldVal"=w475, "NewVal"=w474) -> ("Control out"=w473:refnum<vi>, "P541 Out"=w472:T13)  [unwired: 12 in]
            n216 = Unbundle By Name(w472) -> ("Z Position"=w452:dbl, "Step Size (um)"=w471:dbl)
            n217 = property class="Ctl"(reference=w473) -> ("Label.Text"=w470:string)  [unwired: 1 in, 2 out]
            n218 = call "Manual Controls Action Engine.vi"("Action"=enum16{"Read", "Write"}."Read") -> ("Manual Controls Out"=w461:T18)  [unwired: 14 in]
            n219 = Unbundle By Name(w461) -> ("Z Axis Voltage (I16)"=w464:i16)
            n220 = Multiply(x=w452, y=w453) -> (x*y=w467:dbl)
            n221 = Multiply(x=w471, y=w453) -> (x*y=w469:dbl)
            n222 = Round To Nearest(number=w467) -> (nearest integer value=w456:dbl)
            n223 = Round To Nearest(number=w469) -> (nearest integer value=w455:dbl)
            n224 = To Word Integer(number=w456) -> (16bit integer=w466:i16)
            n225 = To Word Integer(number=w455) -> (16bit integer=w468:i16)
            n226 = case shown="\"Home\"" w470 {
              tunnel: w468 -> [_ w482 w486 _ _ _]
              tunnel: w466 -> [_ _ _ w488 _ _]
              tunnel: w464 -> [w481 w484 w487 _ w493 _]
              tunnel: [w481 w483 w485 w488 w493 w499] -> w460
              tunnel: w453 -> [_ _ _ _ _ w498]
              tunnel: w452 -> [_ _ _ _ w492 _]
              frame Default {
              }
              frame "Step Down" {
                n227 = Subtract(x=w484, y=w482) -> (x-y=w483:i16)
              }
              frame "Step Up" {
                n228 = Add(x=w487, y=w486) -> (x+y=w485:i16)
              }
              frame "Z Position" {
              }
              frame "Save" {
                n229 = Build Array(w492) -> (w491:dbl[])
                n230 = call "Stage_position_ae.vi"("Position In"=w491, "StageID"="P541", "Enum"=enum16{"WRITE", "READ", "HOME", "SAVE HOME"}."SAVE HOME") -> ()  [unwired: 7 in, 2 out]
              }
              frame "Home" {
                n231 = call "Stage_position_ae.vi"("StageID"="P541", "Enum"=enum16{"WRITE", "READ", "HOME", "SAVE HOME"}."HOME") -> ("Position Out"=w496:dbl[])  [unwired: 8 in, 1 out]
                n232 = Index Array(array=w496, index=0) -> (element=w494:dbl)
                n233 = Multiply(x=w494, y=w498) -> (x*y=w500:dbl)
                n234 = Round To Nearest(number=w500) -> (nearest integer value=w501:dbl)
                n235 = To Word Integer(number=w501) -> (16bit integer=w499:i16)
              }
            }
            n236 = Bundle By Name(cluster=w461, "Z Axis Voltage (I16)"=w460) -> (w463:T18)
            n237 = call "Manual Controls Action Engine.vi"("Action"=enum16{"Read", "Write"}."Write", "Manual Controls In"=w463) -> ("Manual Controls Out"=w457:T18)  [unwired: 13 in]
            n238 = call "FPGA-7842R-Control V1.vi"("Action"=FPGA-7842R-Reference."Stage Control", "Manual Controls"=w457, "Initialize"=TRUE) -> ()  [unwired: 11 in, 2 out]
          }
          frame "Phase Comp Mirror - P841" {
            n239 = call "P841_Ctrl_Index.vi"("OldVal"=w516, "NewVal"=w515) -> ("Control out"=w513:refnum<vi>, "P841 Out"=w511:T7)  [unwired: 12 in]
            n240 = property class="Ctl"(reference=w513) -> ("Label.Text"=w512:string)  [unwired: 1 in, 2 out]
            n241 = Unbundle By Name(w511) -> ("Position (µm)"=w510:dbl, "Step Size (µm)"=w509:dbl)
            n242 = case shown="\"Down P841\"" w512 {
              tunnel: w510 -> [_ _ _ w529]
              tunnel: w509 -> [_ w522 w526 _]
              tunnel: [0.0 ("Position (µm)") w522 w525 w529] -> w505
              tunnel: [StageStates."MVR" ("Action") StageStates."MVR" ("Action") StageStates."MVR" ("Action") StageStates."MOVE" ("Action")] -> w508
              tunnel: [enum16{"MOVE", "MVR"}."MVR" ("MOVE/MVR") enum16{"MOVE", "MVR"}."MVR" ("MOVE/MVR") enum16{"MOVE", "MVR"}."MVR" ("MOVE/MVR") enum16{"MOVE", "MVR"}."MOVE" ("MOVE/MVR")] -> w507
              frame Default {
              }
              frame "Up P841" {
              }
              frame "Down P841" {
                n243 = Negate(x=w526) -> (-x=w525:dbl)
              }
              frame "Position (µm)" {
              }
            }
            n244 = Build Array(w505) -> (w504:dbl[])
          }
          frame "Sample Z Coarse - M227" {
            n245 = call "M227_Ctrl_Index.vi"("OldVal"=w545, "NewVal"=w544) -> ("Control Ref OUT"=w543:refnum<vi>, "M227 Out"=w541:T11)  [unwired: 12 in]
            n246 = property class="Ctl"(reference=w543) -> ("Label.Text"=w542:string)  [unwired: 1 in, 2 out]
            n247 = Unbundle By Name(w541) -> ("Step Size (mm)"=w540:dbl, "MM 1"=w533:dbl, "MM 2"=w532:dbl, "MM 3"=w531:dbl)
            n248 = case shown="Default" w542 {
              tunnel: w540 -> [_ _ _ _ w564 w569]
              tunnel: [bool[] [FALSE, FALSE, FALSE] bool[] [TRUE, TRUE, TRUE] bool[] [TRUE, TRUE, TRUE] bool[] [TRUE, TRUE, TRUE] bool[] [TRUE, TRUE, TRUE] bool[] [TRUE, TRUE, TRUE]] -> w538
              tunnel: [0.0 ("Step Size (mm)") w551 w555 w559 w564 w568] -> w535
              tunnel: [StageStates."POSITION" ("Action") StageStates."MOVE" ("Action") StageStates."MOVE" ("Action") StageStates."MOVE" ("Action") StageStates."MVR" ("Action") StageStates."MVR" ("Action")] -> w534
              tunnel: w533 -> [_ w551 _ _ _ _]
              tunnel: w532 -> [_ _ w555 _ _ _]
              tunnel: w531 -> [_ _ _ w559 _ _]
              tunnel: [enum16{"MOVE", "MVR"}."MVR" ("MOVE/MVR") enum16{"MOVE", "MVR"}."MOVE" ("MOVE/MVR") enum16{"MOVE", "MVR"}."MOVE" ("MOVE/MVR") enum16{"MOVE", "MVR"}."MOVE" ("MOVE/MVR") enum16{"MOVE", "MVR"}."MVR" ("MOVE/MVR") enum16{"MOVE", "MVR"}."MVR" ("MOVE/MVR")] -> w530
              frame Default {
              }
              frame "MM 1" {
              }
              frame "MM 2" {
              }
              frame "MM 3" {
              }
              frame "Up M227" {
              }
              frame "Down M227" {
                n249 = Negate(x=w569) -> (-x=w568:dbl)
              }
            }
            n250 = Build Array(w535, w535, w535) -> (w537:dbl[])
          }
        }
        n251 = case shown="\"Cavity Translation Z - ASI\"" w317 {
          frame Default {
          }
          frame "Upper Objective Z - N664" {
            n252 = while {
              i -> [w576]
              stop <- w572 stop-if-true
              n253 = call "Stage_position_ae.vi"("StageID"="N664", "Enum"=enum16{"WRITE", "READ", "HOME", "SAVE HOME"}."READ") -> ("Status Out"=w573:bool, "Position Out"=w583:dbl[])  [unwired: 8 in]
              n254 = Greater?(x=w576, y=200) -> (0:w575:bool)
              n255 = And(x=w573, y=w575) -> (x .and. y?=w572:bool)
              n256 = Wait (ms)(milliseconds to wait=u32 1) -> ()  [unwired: 1 out]
              n257 = Index Array(array=w583, index=0) -> (element=w582:dbl)
              n258 = Select(t=u32 16777215, s=w572, f=u32 6618880) -> (s? t:f=w577:u32)
              n259 = property on="Position (mm)" class="DigNum (strict)"("Value"=w582, "NumText.BG Color"=w577) -> ()  [unwired: 2 in, 2 out]
            }
          }
          frame "Cavity Translation Z - ASI" {
            n260 = while {
              shift-right: [w590] -> _
              shift-left: TRUE ("Status Out") -> [w595]
              stop <- w594 stop-if-true
              n261 = call "Stage_position_ae.vi"("StageID"="ASI", "Enum"=enum16{"WRITE", "READ", "HOME", "SAVE HOME"}."READ") -> ("Status Out"=w590:bool, "Position Out"=w598:dbl[])  [unwired: 8 in]
              n262 = Greater?(x=w590, y=w595) -> (0:w594:bool)
              n263 = Wait (ms)(milliseconds to wait=u32 1) -> ()  [unwired: 1 out]
              n264 = Index Array(array=w598, index=0) -> (element=w588:dbl)
              n265 = Divide(x=w588, y=10.0) -> (x/y=w589:dbl)
              n266 = Select(t=u32 16777215, s=w590, f=u32 6618880) -> (s? t:f=w591:u32)
              n267 = property on="Z (um)" class="DigNum (strict)"("Value"=w589, "NumText.BG Color"=w591) -> ()  [unwired: 2 in, 2 out]
            }
          }
        }
        n268 = control-ref of="Abort AllStage"() -> (w308:refnum<vi>)
        n269 = call "AllStage_Limits_Array.vi"("Step(um)/Position(units)"=w315, "Axis"=w314, "Stage ID"=w316, "MOVE/MVR"=w313) -> ("Positions"=w311:dbl[], "Boolean Array"=w310:bool[], "Stage ID"=w312:string)  [unwired: 5 in]
        n270 = call "AE_AllStages_Action V2.vi"("Velocity"=w309, "Abort"=w308, "Positions"=w311, "Axis"=w310, "Stage ID"=w312, "Action"=w307) -> ()  [unwired: 3 in, 3 out]
      }
      event "SLM", "Timing", "DM", "Camera": Value Change {
        n271 = event-data() -> ("CtlRef"=w603:refnum<vi>, "NewVal"=w600:bool)  [unwired: 1 in, 1 out]
        n272 = property class="Bool (strict)"(reference=w603) -> ("Label.Text"=w602:string)  [unwired: 1 in, 2 out]
        n273 = case shown="\"Timing\"" w602 {
          tunnel: w600 -> [w604 w618 w632 w646 w659]
          frame "SLM", Default {
            n274 = case shown="True" w604 {
              frame False {
                n275 = To Variant(anything=TRUE) -> (Variant=w610:variant)
                n276 = call "SLM AE.vi"("Action"=enum16{"READ", "WRITE"}."READ") -> ("SLM Ref Out"=w611:refnum<vi>)  [unwired: 10 in]
                n277 = invoke class="VI" method="Ctrl Val.Set"(reference=w611, "Control Name"="Exit", "Value"=w610) -> (reference out=w607:refnum<vi>, error out=w606:errorcluster)  [unwired: 2 in, 3 out]
                n278 = invoke on="Hamamatsu LCOS" class="SubPnl" method="Remove VI"(error in=w606) -> (error out=w605:errorcluster)  [unwired: 2 in, 2 out]
                n279 = Close Reference(reference=w607, error in (no error)=w605) -> ()  [unwired: 1 out]
              }
              frame True {
                n280 = Open VI Reference(vi path=path "C:/Users/ED STED/Documents/Test Control Software/Host VIs/SLM_V2/SLM Control.vi") -> (vi reference=w616:refnum<vi>)  [unwired: 5 in, 1 out]
                n281 = invoke class="VI" method="Run VI"(reference=w616, "Wait until done"=FALSE ("Wait Until Done")) -> (reference out=w613:refnum<vi>)  [unwired: 3 in, 4 out]
                n282 = invoke on="Hamamatsu LCOS" class="SubPanel" method="Insert VI"("VI Ref"=w613) -> ()  [unwired: 3 in, 4 out]
                n283 = call "SLM AE.vi"("Action"=enum16{"READ", "WRITE"}."WRITE", "SLM Ref In"=w613) -> ()  [unwired: 9 in, 1 out]
              }
            }
          }
          frame "DM" {
            n284 = case shown="False" w618 {
              frame False {
                n285 = call "DM_Ref_AE.vi"("Action"=enum16{"READ", "WRITE"}."READ") -> ("DM Ref Out"=w625:refnum<vi>)  [unwired: 10 in]
                n286 = To Variant(anything=TRUE) -> (Variant=w624:variant)
                n287 = invoke class="VI" method="Ctrl Val.Set"(reference=w625, "Control Name"="Exit", "Value"=w624) -> (reference out=w621:refnum<vi>, error out=w620:errorcluster)  [unwired: 2 in, 3 out]
                n288 = invoke on="BM Multi" class="SubPnl" method="Remove VI"(error in=w620) -> (error out=w619:errorcluster)  [unwired: 2 in, 2 out]
                n289 = Close Reference(reference=w621, error in (no error)=w619) -> ()  [unwired: 1 out]
              }
              frame True {
                n290 = Open VI Reference(vi path=path "C:/Users/ED STED/Documents/Test Control Software/Host VIs/DM_Dual_V2/Dual_DM_Control_Main_V3.vi") -> (vi reference=w630:refnum<vi>)  [unwired: 5 in, 1 out]
                n291 = invoke class="VI" method="Run VI"(reference=w630, "Wait until done"=FALSE ("Wait Until Done")) -> (reference out=w627:refnum<vi>)  [unwired: 3 in, 4 out]
                n292 = invoke on="BM Multi" class="SubPanel" method="Insert VI"("VI Ref"=w627) -> ()  [unwired: 3 in, 4 out]
                n293 = call "DM_Ref_AE.vi"("Action"=enum16{"READ", "WRITE"}."WRITE", "DM Ref In"=w627) -> ()  [unwired: 9 in, 1 out]
              }
            }
          }
          frame "Timing" {
            n294 = case shown="True" w632 {
              frame False {
                n295 = To Variant(anything=TRUE) -> (Variant=w637:variant)
                n296 = call "GateDelay AE.vi"("Action"=enum16{"READ", "WRITE"}."READ") -> ("Gate Delay Ref Out"=w638:refnum<vi>)  [unwired: 10 in]
                n297 = invoke class="VI" method="Ctrl Val.Set"(reference=w638, "Control Name"="Exit", "Value"=w637) -> (reference out=w633:refnum<vi>, error out=w634:errorcluster)  [unwired: 2 in, 3 out]
                n298 = invoke on="Timing" class="SubPnl" method="Remove VI"(error in=w634) -> (error out=w640:errorcluster)  [unwired: 2 in, 2 out]
                n299 = Close Reference(reference=w633, error in (no error)=w640) -> ()  [unwired: 1 out]
              }
              frame True {
                n300 = Open VI Reference(vi path=path "C:/Users/ED STED/Documents/Test Control Software/Host VIs/Time Delay/GateDelay_Control_V2.vi") -> (vi reference=w643:refnum<vi>)  [unwired: 5 in, 1 out]
                n301 = invoke class="VI" method="Run VI"(reference=w643, "Wait until done"=FALSE ("Wait Until Done")) -> (reference out=w642:refnum<vi>)  [unwired: 3 in, 4 out]
                n302 = invoke on="Timing" class="SubPanel" method="Insert VI"("VI Ref"=w642) -> ()  [unwired: 3 in, 4 out]
                n303 = call "GateDelay AE.vi"("Action"=enum16{"READ", "WRITE"}."WRITE", "Gate Delay Ref In"=w642) -> ()  [unwired: 9 in, 1 out]
              }
            }
          }
          frame "Camera" {
            n304 = case shown="True" w646 {
              frame False {
                n305 = To Variant(anything=TRUE) -> (Variant=w647:variant)
                n306 = call "Camera_Ref_HX.vi"("Action"=enum16{"READ", "WRITE"}."READ") -> ("Alignment Ref Out"=w651:refnum<vi>)  [unwired: 10 in]
                n307 = invoke class="VI" method="Ctrl Val.Set"(reference=w651, "Control Name"="Exit", "Value"=w647) -> (reference out=w650:refnum<vi>)  [unwired: 2 in, 4 out]
                n308 = invoke on="uc480" class="SubPnl" method="Remove VI"() -> (error out=w652:errorcluster)  [unwired: 3 in, 2 out]
                n309 = Close Reference(reference=w650, error in (no error)=w652) -> ()  [unwired: 1 out]
              }
              frame True {
                n310 = Open VI Reference(vi path=path "C:/Users/ED STED/Documents/Test Control Software/Host VIs/Camera/uEye_Control_V1.vi") -> (vi reference=w656:refnum<vi>)  [unwired: 5 in, 1 out]
                n311 = invoke class="VI" method="Run VI"(reference=w656, "Wait until done"=FALSE ("Wait Until Done")) -> (reference out=w655:refnum<vi>)  [unwired: 3 in, 4 out]
                n312 = invoke on="uc480" class="SubPnl" method="Insert VI"("VI Ref"=w655) -> ()  [unwired: 3 in, 4 out]
                n313 = call "Camera_Ref_HX.vi"("Action"=enum16{"READ", "WRITE"}."WRITE", "Alignment Ref In"=w655) -> ()  [unwired: 9 in, 1 out]
              }
            }
          }
          frame "Alignment" {
            n314 = case shown="True" w659 {
              frame False {
                n315 = To Variant(anything=TRUE) -> (Variant=w660:variant)
                n316 = call "FocusLock_Ref_HX.vi"("Action"=enum16{"READ", "WRITE"}."READ") -> ("Camera Ref Out"=w664:refnum<vi>)  [unwired: 10 in]
                n317 = invoke class="VI" method="Ctrl Val.Set"(reference=w664, "Control Name"="Exit", "Value"=w660) -> (reference out=w663:refnum<vi>)  [unwired: 2 in, 4 out]
                n318 = invoke on="uc480" class="SubPnl" method="Remove VI"() -> (error out=w665:errorcluster)  [unwired: 3 in, 2 out]
                n319 = Close Reference(reference=w663, error in (no error)=w665) -> ()  [unwired: 1 out]
              }
              frame True {
                n320 = Open VI Reference(vi path=path "C:/Users/ED STED/Documents/Test Control Software/Host VIs/AutoAlign/AutoAlign_SWITCH.vi") -> (vi reference=w669:refnum<vi>)  [unwired: 5 in, 1 out]
                n321 = invoke class="VI" method="Run VI"(reference=w669, "Wait until done"=FALSE ("Wait Until Done")) -> (reference out=w668:refnum<vi>)  [unwired: 3 in, 4 out]
                n322 = invoke on="uc480" class="SubPnl" method="Insert VI"("VI Ref"=w668) -> ()  [unwired: 3 in, 4 out]
                n323 = call "FocusLock_Ref_HX.vi"("Action"=enum16{"READ", "WRITE"}."WRITE", "Camera Ref In"=w668) -> ()  [unwired: 9 in, 1 out]
              }
            }
          }
        }
      }
      event Value Change {
        n324 = event-data() -> ("CtlRef"=w677:refnum<vi>, "OldVal"=w675:variant, "NewVal"=w674:variant)  [unwired: 1 in]
        n325 = property class="Clust"(reference=w677) -> ("Label.Text"=w676:string)  [unwired: 1 in, 2 out]
        n326 = call "Graph Ref AE.vi"("Action"=enum16{"READ", "WRITE"}."READ") -> ("Graph Ref Out"=w672:refnum<vi>[])  [unwired: 10 in]
        n327 = case shown="\"Graph Tools\"" w676 {
          tunnel: w675 -> [_ w684 w740]
          tunnel: w674 -> [_ w685 w739]
          tunnel: w672 -> [_ w679 w732]
          frame Default {
          }
          frame "Display Controls" {
            n328 = call "Display_Controls_Ctrl_Index.vi"("OldVal"=w684, "NewVal"=w685) -> ("Control Ref OUT"=w683:refnum<vi>, "Display Controls Out"=w681:T2)  [unwired: 12 in]
            n329 = property class="Ctl"(reference=w683) -> ("Label.Text"=w682:string)  [unwired: 1 in, 2 out]
            n330 = Unbundle By Name(w681) -> ("Single Screen"=w680:bool)
            n331 = case shown="\"Single Screen\", Default" w682 {
              tunnel: w680 -> [w693 _ _]
              tunnel: w679 -> [_ w718 w725]
              frame "Single Screen", Default {
                n332 = property class="App"() -> ("Disp.AllMonitors"=w692:T31)  [unwired: 2 in, 2 out]
                n333 = Index Array(array=w692, index #1=2 ("index"), index #2=0 ("index")) -> (element #1=w689:T32, element #2=w688:T32)
                n334 = control-ref of="This VI"() -> (w687:refnum<vi>)
                n335 = case shown="False" w693 {
                  tunnel: w689 -> [w697 _]
                  tunnel: w688 -> [w696 w708]
                  tunnel: w687 -> [w695 w706]
                  tunnel: T22 {"Left"=0, "Top"=0, "Right"=0, "Bottom"=0} ("Front Panel Window:Window Bounds") -> [w694 w707]
                  frame False {
                    w702 = i16 0
                    n336 = Unbundle By Name(w696) -> ("Bounds.Left"=w699:i16, "Bounds.Bottom"=w700:i16, "Bounds.Top"=w701:i16)
                    n337 = Unbundle By Name(w697) -> ("Bounds.Right"=w698:i16)
                    n338 = Subtract(x=w698, y=w699) -> (x-y=w703:i16)
                    n339 = Subtract(x=w700, y=w701) -> (x-y=w704:i16)
                    n340 = Bundle By Name(cluster=w694, "Left"=w702, "Top"=w702, "Right"=w703, "Bottom"=w704) -> (w705:T22)
                    n341 = property class="VI"(reference=w695, "Front Panel.WinBounds"=w705) -> ()  [unwired: 1 in, 2 out]
                  }
                  frame True {
                    w711 = i16 0
                    n342 = Unbundle By Name(w708) -> ("Bounds.Right"=w714:i16, "Bounds.Bottom"=w713:i16, "Bounds.Top"=w712:i16)
                    n343 = Subtract(x=w713, y=w712) -> (x-y=w710:i16)
                    n344 = Bundle By Name(cluster=w707, "Left"=w711, "Top"=w711, "Right"=w714, "Bottom"=w710) -> (w709:T22)
                    n345 = property class="VI"(reference=w706, "Front Panel.WinBounds"=w709) -> (reference out=w716:refnum<vi>)  [unwired: 1 in, 1 out]
                    n346 = property class="VI"(reference=w716, "FP.State"=T23."Maximized" ("Front Panel Window:State")) -> ()  [unwired: 1 in, 2 out]
                  }
                }
              }
              frame "Add Display" {
                w719 = u16 0 items=["Read", "Write"] ("Action")
                w723 = u16 1 items=["Read", "Write"] ("Action")
                n347 = property on="Add Display" class="Bool (strict)"("Value"=FALSE) -> ()  [unwired: 2 in, 2 out]
                n348 = call "Arange_Displays_V2.vi"("Action"=w719) -> ("Number of Channels OUT"=w720:i32)  [unwired: 14 in]
                n349 = Increment(x=w720) -> (x+1=w722:i32)
                n350 = call "Arange_Displays_V2.vi"("Display References"=w718, "Action"=w723, "Number of Channels"=w722, "Aspect Ratio (h/w)"=1.0) -> ()  [unwired: 11 in, 1 out]
              }
              frame "Remove Display" {
                w726 = u16 0 items=["Read", "Write"] ("Action")
                w730 = u16 1 items=["Read", "Write"] ("Action")
                n351 = call "Arange_Displays_V2.vi"("Action"=w726) -> ("Number of Channels OUT"=w727:i32)  [unwired: 14 in]
                n352 = Decrement(x=w727) -> (x-1=w729:i32)
                n353 = call "Arange_Displays_V2.vi"("Display References"=w725, "Action"=w730, "Number of Channels"=w729, "Aspect Ratio (h/w)"=1.0) -> ()  [unwired: 11 in, 1 out]
                n354 = property on="Remove Display" class="Bool (strict)"("Value"=FALSE) -> ()  [unwired: 2 in, 2 out]
              }
            }
          }
          frame "Graph Tools" {
            n355 = call "Graph_Controls_Ctrl_Index.vi"("OldVal"=w740, "NewVal"=w739) -> ("Control Ref OUT"=w738:refnum<vi>, "Graph Tools Out"=w737:T3)  [unwired: 12 in]
            n356 = property class="Ctl"(reference=w738) -> (reference out=w734:refnum<vi>, "Label.Text"=w733:string)  [unwired: 1 in, 1 out]
            n357 = Unbundle By Name(w737) -> ("Show Cursor"=w736:bool, "Auto Scale"=w735:bool, "Color Map"=w731:T33)
            n358 = case shown="\"Apply Color\"" w733 {
              selector: w733 -> [_ _ _ w809 _ _ _ _]
              tunnel: w736 -> [_ w778 _ _ _ _ _ _]
              tunnel: w735 -> [_ _ w798 _ _ _ _ _]
              tunnel: w732 -> [w749 w777 w799 w802 w839 _ w851 w859]
              tunnel: w734 -> [_ _ _ _ _ _ _ _]
              tunnel: w733 -> [_ _ _ w804 _ _ _ _]
              tunnel: w731 -> [w752 _ _ _ _ _ _ _]
              frame "Apply Color" {
                n359 = control-ref of="This VI"() -> (w751:refnum<vi>)
                n360 = call "GetDisplayClick.vi"("Display REFs In"=w749, "Calling VI REF"=w751) -> ("Display Index"=w750:i32)  [unwired: 13 in]
                n361 = Index Array(array=w749, index=w750) -> (element=w748:refnum<vi>)
                n362 = property class="IntGraph (strict)"(reference=w748) -> (reference out=w744:refnum<vi>, error out=w741:errorcluster, "ZScale.Maximum"=w747:dbl)  [unwired: 1 in]
                n363 = case shown="\"Gray\"" w752 {
                  tunnel: [cluster{dbl, u32}[] [{0.0, 0}, {85.0, 16711680}, {108.0, 16729344}, {127.0, 16744192}, {132.0, 16747520}, {140.0, 16753920}, {157.0, 16766720}, {170.0, 16776960}, {245.0, 16777184}, {250.0, 16777200}, {255.0, 16777215}] ("Z Scale.Marker Values[]") cluster{dbl, u32}[] [{0.0, 0}, {255.0, 16777215}] ("Z Scale.Marker Values[]") cluster{dbl, u32}[] [{0.0, 0}, {255.0, 16711680}] ("Z Scale.Marker Values[]") cluster{dbl, u32}[] [{0.0, 0}, {255.0, 65280}] ("Z Scale.Marker Values[]") cluster{dbl, u32}[] [{0.0, 0}, {255.0, 255}] ("Z Scale.Marker Values[]") cluster{dbl, u32}[] [{0.0, 0}, {255.0, 65535}] ("Z Scale.Marker Values[]") cluster{dbl, u32}[] [{0.0, 0}, {255.0, 16711935}] ("Z Scale.Marker Values[]") cluster{dbl, u32}[] [{0.0, 0}, {255.0, 16776960}] ("Z Scale.Marker Values[]") cluster{dbl, u32}[] [{0.0, 0}, {170.0, 16711680}, {245.0, 16777184}, {250.0, 16777200}, {255.0, 16448250}] ("Z Scale.Marker Values[]") cluster{dbl, u32}[] [{0.0, 0}, {170.0, 65280}, {245.0, 16777184}, {250.0, 16777200}, {255.0, 16448250}] ("Z Scale.Marker Values[]") cluster{dbl, u32}[] [{0.0, 0}, {170.0, 255}, {245.0, 16777184}, {250.0, 16777200}, {255.0, 16448250}] ("Z Scale.Marker Values[]") cluster{dbl, u32}[] [{0.0, 0}, {1.0, 131072}, {2.0, 196608}, {3.0, 327680}, {4.0, 458752}, {5.0, 589824}, {6.0, 720896}, {7.0, 851971}, {8.0, 983043}, {9.0, 1114115}, {10.0, 1245187}, {11.0, 1376259}, {12.0, 1507331}, {13.0, 1638403}, {14.0, 1769475}, {15.0, 1769479}, {16.0, 2031623}, {17.0, 2162695}, {18.0, 2293767}, {19.0, 2424839}, {20.0, 2555911}, {21.0, 2686983}, {22.0, 2818055}, {23.0, 2949127}, {24.0, 3080203}, {25.0, 3211275}, {26.0, 3342347}, {27.0, 3473419}, {28.0, 3604491}, {29.0, 3735563}, {30.0, 3866635}, {31.0, 3867403}, {32.0, 4129547}, {33.0, 4260619}, {34.0, 4391691}, {35.0, 4522763}, {36.0, 4653839}, {37.0, 4784911}, {38.0, 4915983}, {39.0, 5178127}, {40.0, 5309199}, {41.0, 5440271}, {42.0, 5571343}, {43.0, 5702415}, {44.0, 5703439}, {45.0, 5965583}, {46.0, 6096655}, {47.0, 6227727}, {48.0, 6358799}, {49.0, 6489871}, {50.0, 6620943}, {51.0, 6752015}, {52.0, 6883087}, {53.0, 7015183}, {54.0, 7146255}, {55.0, 7277327}, {56.0, 7408399}, {57.0, 7539471}, {58.0, 7670543}, {59.0, 7801615}, {60.0, 8063759}, {61.0, 8194831}, {62.0, 8326927}, {63.0, 8457999}, {64.0, 8589075}, {65.0, 8720147}, {66.0, 8851219}, {67.0, 8982291}, {68.0, 9113363}, {69.0, 9114387}, {70.0, 9376531}, {71.0, 9507603}, {72.0, 9638675}, {73.0, 9769747}, {74.0, 9901843}, {75.0, 10032915}, {76.0, 10163987}, {77.0, 10229523}, {78.0, 10295059}, {79.0, 10427155}, {80.0, 10558227}, {81.0, 10689299}, {82.0, 10820371}, {83.0, 10886931}, {84.0, 10952467}, {85.0, 11083539}, {86.0, 11214611}, {87.0, 11215635}, {88.0, 11477779}, {89.0, 11543315}, {90.0, 11608851}, {91.0, 11740947}, {92.0, 11806483}, {93.0, 11872019}, {94.0, 12004115}, {95.0, 12135187}, {96.0, 12266259}, {97.0, 12267283}, {98.0, 12398355}, {99.0, 12529427}, {100.0, 12530451}, {101.0, 12595987}, {102.0, 12530451}, {103.0, 12793619}, {104.0, 12794131}, {105.0, 12794643}, {106.0, 13056787}, {107.0, 13057299}, {108.0, 13057811}, {109.0, 13188883}, {110.0, 13320979}, {111.0, 13386515}, {112.0, 13452563}, {113.0, 13584147}, {114.0, 13584659}, {115.0, 13585171}, {116.0, 13585683}, {117.0, 13717267}, {118.0, 13848339}, {119.0, 13849363}, {120.0, 13849875}, {121.0, 13850387}, {122.0, 13981459}, {123.0, 14113555}, {124.0, 14114067}, {125.0, 14114579}, {126.0, 14115091}, {127.0, 14246675}, {128.0, 14377747}, {129.0, 14378771}, {130.0, 14379283}, {131.0, 14379539}, {132.0, 14379795}, {133.0, 14380819}, {134.0, 14511891}, {135.0, 14643987}, {136.0, 14644503}, {137.0, 14645015}, {138.0, 14645527}, {139.0, 14646039}, {140.0, 14646551}, {141.0, 14778135}, {142.0, 14909207}, {143.0, 14910231}, {144.0, 14910747}, {145.0, 14911259}, {146.0, 14911771}, {147.0, 14912283}, {148.0, 14912797}, {149.0, 15044383}, {150.0, 15175455}, {151.0, 15175967}, {152.0, 15176479}, {153.0, 15176991}, {154.0, 15177507}, {155.0, 15178019}, {156.0, 15178531}, {157.0, 15310115}, {158.0, 15441701}, {159.0, 15441959}, {160.0, 15442215}, {161.0, 15442727}, {162.0, 15443243}, {163.0, 15443755}, {164.0, 15444269}, {165.0, 15444783}, {166.0, 15444783}, {167.0, 15576367}, {168.0, 15707953}, {169.0, 15708467}, {170.0, 15708979}, {171.0, 15708981}, {172.0, 15708983}, {173.0, 15710011}, {174.0, 15710523}, {175.0, 15711037}, {176.0, 15711039}, {177.0, 15711553}, {178.0, 15843139}, {179.0, 15974213}, {180.0, 15974215}, {181.0, 15974217}, {182.0, 15974219}, {183.0, 15975755}, {184.0, 15976271}, {185.0, 15976785}, {186.0, 15977299}, {187.0, 15977301}, {188.0, 15977815}, {189.0, 15978327}, {190.0, 15978331}, {191.0, 16109917}, {192.0, 16241503}, {193.0, 16241505}, {194.0, 16242019}, {195.0, 16242535}, {196.0, 16242537}, {197.0, 16242539}, {198.0, 16243563}, {199.0, 16243567}, {200.0, 16244081}, {201.0, 16244595}, {202.0, 16244599}, {203.0, 16244601}, {204.0, 16244603}, {205.0, 16245627}, {206.0, 16245631}, {207.0, 16245633}, {208.0, 16246147}, {209.0, 16246663}, {210.0, 16377735}, {211.0, 16508811}, {212.0, 16508815}, {213.0, 16509839}, {214.0, 16509843}, {215.0, 16509845}, {216.0, 16509847}, {217.0, 16510361}, {218.0, 16510875}, {219.0, 16510879}, {220.0, 16510881}, {221.0, 16510883}, {222.0, 16511399}, {223.0, 16511911}, {224.0, 16511915}, {225.0, 16511917}, {226.0, 16511919}, {227.0, 16511923}, {228.0, 16512437}, {229.0, 16512951}, {230.0, 16512955}, {231.0, 16512957}, {232.0, 16512959}, {233.0, 16512961}, {234.0, 16512963}, {235.0, 16512967}, {236.0, 16513481}, {237.0, 16513995}, {238.0, 16513999}, {239.0, 16514001}, {240.0, 16514003}, {241.0, 16514005}, {242.0, 16514007}, {243.0, 16514011}, {244.0, 16514013}, {245.0, 16514015}, {246.0, 16514019}, {247.0, 16514021}, {248.0, 16514023}, {249.0, 16514027}, {250.0, 16514029}, {251.0, 16514031}, {252.0, 16514035}, {253.0, 16514037}, {254.0, 16514039}, {255.0, 16514043}] ("Z Scale.Marker Values[]")] -> w743
                  tunnel: w747 -> [w753 w755 w757 w759 w761 w763 w765 w767 w769 w771 w773 w776]
                  tunnel: [w753 w755 w757 w759 w761 w763 w765 w767 w769 w771 w773 w776] -> w745
                  frame "Fire", Default {
                    # "Fire"
                  }
                  frame "Gray" {
                    # "Grayscale"
                  }
                  frame "Red" {
                    # "Red"
                  }
                  frame "Green" {
                    # "Green"
                  }
                  frame "Blue" {
                    # "Blue"
                  }
                  frame "Cyan" {
                    # "Cyan"
                  }
                  frame "Magenta" {
                    # "Magenta"
                  }
                  frame "Yellow" {
                    # "Yellow"
                  }
                  frame "Red-White" {
                    # "Red-White"
                  }
                  frame "Green-White" {
                    # "Green-White"
                  }
                  frame "Blue-White" {
                    # "Blue-White"
                  }
                  frame "Glow" {
                  }
                }
                n364 = property on="Apply Color" class="Bool (strict)"(error in=w741, "Value"=FALSE) -> ()  [unwired: 1 in, 2 out]
                n365 = property class="IntGraph (strict)"(reference=w744, "ZScale.MarkerVals[]"=w743, "ZScale.High Color"=u32 255, "ZScale.Maximum"=w745) -> ()  [unwired: 1 in, 2 out]
              }
              frame "Show Cursor", Default {
                w781 = 2.0 ("y")
                n366 = Index Array(array=w777, index=0) -> (element=w789:refnum<vi>)
                n367 = property class="IntGraph (strict)"(reference=w789) -> ("Value"=w788:sgl[][])  [unwired: 1 in, 2 out]
                n368 = Array Size(array=w788) -> (size(s)=w787:i32[])
                n369 = To Double Precision Float(number=w787) -> (double precision float=w784:dbl[])
                n370 = Index Array(array=w784, index #1=0 ("index"), index #2=1 ("index")) -> (element #1=w783:dbl, element #2=w782:dbl)
                n371 = Divide(x=w783, y=w781) -> (x/y=w780:dbl)
                n372 = Divide(x=w782, y=w781) -> (x/y=w779:dbl)
                n373 = for {
                  tunnel: w777 -> [w791] mode=indexing
                  tunnel: w780 -> [w793]
                  tunnel: w779 -> [w792]
                  tunnel: w778 -> [w794]
                  n374 = property class="IntGraph (strict)"(reference=w791, "Cursor.Visible"=w794, "Cursor.Cursor X"=w793, "Cursor.Cursor Y"=w792) -> ()  [unwired: 1 in, 2 out]
                }
              }
              frame "Auto Scale" {
                n375 = Select(t=u8 2 ("Z Scale.Scale Fit"), s=w798, f=u8 0) -> (s? t:f=w795:u8)
                n376 = for {
                  tunnel: w799 -> [w801] mode=indexing
                  tunnel: w795 -> [w800]
                  n377 = property class="IntGraph (strict)"(reference=w801, "ZScale.ScaleFit"=w800) -> ()  [unwired: 1 in, 2 out]
                }
              }
              frame "Pan Tool", "Reset Zoom", "Zoom In", "Zoom Out" {
                n378 = case shown="\"Reset Zoom\"" w809 {
                  tunnel: [0 ("Palette:Active Tool") 6 ("Palette:Active Tool") 7 ("Palette:Active Tool") 1 ("Palette:Active Tool") 0 ("Palette:Active Tool")] -> w803
                  tunnel: w802 -> [_ _ _ _ w821]
                  frame Default {
                  }
                  frame "Zoom In" {
                  }
                  frame "Zoom Out" {
                  }
                  frame "Pan Tool" {
                  }
                  frame "Reset Zoom" {
                    n379 = property on="Reset Zoom" class="Bool (strict)"("Value"=FALSE) -> ()  [unwired: 2 in, 2 out]
                    n380 = for {
                      tunnel: w821 -> [w826] mode=indexing
                      tunnel: 5 ("Palette:Active Tool") -> [w825]
                      n381 = property class="IntGraph (strict)"(reference=w826, "ActPaletteTool"=w825) -> ()  [unwired: 1 in, 2 out]
                    }
                  }
                }
                n382 = control-ref of="Zoom In"() -> (w805:refnum<vi>)
                n383 = control-ref of="Zoom Out"() -> (w807:refnum<vi>)
                n384 = control-ref of="Pan Tool"() -> (w806:refnum<vi>)
                n385 = Build Array(w805, w807, w806) -> (w808:refnum<vi>[])
                n386 = for {
                  tunnel: w808 -> [w814] mode=indexing
                  tunnel: w804 -> [w812]
                  n387 = property class="Bool (strict)"(reference=w814) -> (reference out=w813:refnum<vi>, "Label.Text"=w811:string)  [unwired: 1 in, 1 out]
                  n388 = Equal?(x=w811, y=w812) -> (x = y?=w810:bool)
                  n389 = property class="Bool (strict)"(reference=w813, "Value"=w810) -> ()  [unwired: 1 in, 2 out]
                }
                n390 = for {
                  tunnel: w802 -> [w816] mode=indexing
                  tunnel: w803 -> [w815]
                  n391 = property class="IntGraph (strict)"(reference=w816, "ActPaletteTool"=w815) -> ()  [unwired: 1 in, 2 out]
                }
              }
              frame "Load File" {
                w836 = u16 1 items=["Get Image", "Load and Read File"] ("Action")
                n392 = control-ref of="This VI"() -> (w838:refnum<vi>)
                n393 = property on="Load File" class="Bool (strict)"("Value"=FALSE) -> ()  [unwired: 2 in, 2 out]
                n394 = call "GetDisplayClick.vi"("Display REFs In"=w839, "Calling VI REF"=w838) -> ("Display Index"=w827:i32)  [unwired: 13 in]
                n395 = call "OpenDBL.vi"("Action"=w836) -> ("Image"=w835:sgl[], "Dimensions (Z, Y, X, t)"=w834:i32[])  [unwired: 11 in, 2 out]
                n396 = Index Array(array=w834, index #1=1 ("index"), index #2=2 ("index")) -> (element #1=w831:i32, element #2=w830:i32)
                n397 = Reverse 1D Array(array=w835) -> (reversed array=w829:sgl[])
                n398 = Reshape Array(w829, w831, w830) -> (w828:sgl[][])
                n399 = Index Array(array=w839, index=w827) -> (element=w837:refnum<vi>)
                n400 = property class="IntGraph (strict)"(reference=w837, "Value"=w828) -> ()  [unwired: 1 in, 2 out]
              }
              frame "Fit Tool" {
                n401 = disable-structure shown="Disabled" {
                  frame Disabled {
                    n402 = vi-ref "QuickProfile_V4.vi"() -> (w843:refnum<vi>)
                    n403 = call "Image Aquisition Param Ctrl_AE.vi"("Action"=enum16{"READ", "WRITE"}."READ") -> ()  [unwired: 10 in, 1 out]
                    n404 = property class="VI Interface Type 0"(reference=w843) -> ("Path"=w846:path)  [unwired: 1 in, 2 out]
                    n405 = Unbundle By Name() -> ("Pixel Size (nm)"=w842:dbl[])  [unwired: 1 in]
                    n406 = Index Array(array=w842, index=0) -> (element=w849:dbl)
                    n407 = Open VI Reference(type specifier VI Refnum (for type only)=w843, vi path=w846, options=128) -> (vi reference=w844:refnum<vi>)  [unwired: 3 in, 1 out]
                    n408 = call-by-ref "Start Asynchronous Call"(reference=w844, "Pixel Size (nm)"=w849) -> (reference out=w847:refnum<vi>)  [unwired: 16 in, 1 out]
                    n409 = Close Reference(reference=w847) -> ()  [unwired: 1 in, 1 out]
                  }
                  frame Enabled {
                  }
                }
              }
              frame "Smooth Tool" {
                n410 = vi-ref "SmoothTool.vi"() -> (w854:refnum<vi>)
                n411 = property on="Smooth Tool" class="Bool (strict)"("Value"=FALSE) -> ()  [unwired: 2 in, 2 out]
                n412 = property class="VI Interface Type 1"(reference=w854) -> ("Path"=w856:path)  [unwired: 1 in, 2 out]
                n413 = control-ref of="This VI"() -> (w852:refnum<vi>)
                n414 = Open VI Reference(type specifier VI Refnum (for type only)=w854, vi path=w856, options=128) -> (vi reference=w855:refnum<vi>)  [unwired: 3 in, 1 out]
                n415 = call-by-ref "Start Asynchronous Call"(reference=w855, "Calling VI REF"=w852, "Display REFs In"=w851) -> (reference out=w853:refnum<vi>)  [unwired: 11 in, 1 out]
                n416 = Close Reference(reference=w853) -> ()  [unwired: 1 in, 1 out]
              }
              frame "Merge Tool" {
                n417 = vi-ref "MergeTool - Cambridge.vi"() -> (w862:refnum<vi>)
                n418 = property class="VI Interface Type 2"(reference=w862) -> ("Path"=w864:path)  [unwired: 1 in, 2 out]
                n419 = property on="Merge Tool" class="Bool (strict)"("Value"=FALSE) -> ()  [unwired: 2 in, 2 out]
                n420 = control-ref of="This VI"() -> (w860:refnum<vi>)
                n421 = Open VI Reference(type specifier VI Refnum (for type only)=w862, vi path=w864, options=128) -> (vi reference=w863:refnum<vi>)  [unwired: 3 in, 1 out]
                n422 = call-by-ref "Start Asynchronous Call"(reference=w863, "VI Reference"=w860, "Display References"=w859) -> (reference out=w861:refnum<vi>)  [unwired: 11 in, 1 out]
                n423 = Close Reference(reference=w861) -> ()  [unwired: 1 in, 1 out]
              }
            }
          }
        }
      }
      event "Channel 1", "Channel 2", "Channel 3", "Channel 4", "Channel 5", "Channel 6": Mouse Down; "Channel 1", "Channel 2", "Channel 3", "Channel 4", "Channel 5", "Channel 6": Mouse Up {
        n424 = event-data() -> ("Type"=w871:T24, "CtlRef"=w868:refnum<vi>)  [unwired: 1 in, 5 out]
        n425 = Equal?(x=w871, y=lveventtype."Mouse Down" ("Type")) -> (x = y?=w869:bool)
        n426 = call "Graph Ref AE.vi"("Action"=enum16{"READ", "WRITE"}."READ") -> ("Graph Ref Out"=w866:refnum<vi>[])  [unwired: 10 in]
        n427 = case shown="True" w869 {
          tunnel: w868 -> [w874 w892]
          tunnel: w866 -> [w873 w891]
          frame False {
            n428 = property class="IntGraph (strict)"(reference=w874) -> (reference out=w878:refnum<vi>, "ActPaletteTool"=w875:i32)  [unwired: 1 in, 1 out]
            n429 = Not Equal?(x=w875, y=0) -> (x != y?=w877:bool)
            n430 = case shown="False" w877 {
              tunnel: w878 -> [w881 w887]
              tunnel: w873 -> [w880 w884]
              frame False {
                n431 = property class="IntGraph (strict)"(reference=w881) -> ("Cursor.Cursor Position"=w879:T34)  [unwired: 1 in, 2 out]
                n432 = for {
                  tunnel: w880 -> [w882] mode=indexing
                  tunnel: w879 -> [w883]
                  n433 = property class="IntGraph (strict)"(reference=w882, "Cursor.Cursor Position"=w883) -> ()  [unwired: 1 in, 2 out]
                }
              }
              frame True {
                n434 = property class="IntGraph (strict)"(reference=w887) -> ("XScale.Range"=w886:T35, "YScale.Range"=w885:T35)  [unwired: 1 in, 2 out]
                n435 = for {
                  tunnel: w886 -> [w890]
                  tunnel: w885 -> [w889]
                  tunnel: w884 -> [w888] mode=indexing
                  n436 = property class="IntGraph (strict)"(reference=w888, "XScale.Range"=w890, "YScale.Range"=w889) -> ()  [unwired: 1 in, 2 out]
                }
              }
            }
          }
          frame True {
            n437 = for {
              tunnel: w891 -> [w897] mode=indexing
              tunnel: w892 -> [w898]
              n438 = Equal?(x=w897, y=w898) -> (x = y?=w896:bool)
              n439 = Select(t=T25 {"Left"=2431, "Top"=-324} ("Z Scale.Position"), s=w896, f=T25 {"Left"=0, "Top"=0}) -> (s? t:f=w893:T25)
              n440 = property class="IntGraph (strict)"(reference=w897, "ZScale.Visible"=w896, "ZScale.Position"=w893) -> ()  [unwired: 1 in, 2 out]
            }
          }
        }
      }
      event "Exit": Value Change {
        n441 = event-data() -> ("CtlRef"=w923:refnum<vi>, "NewVal"=w925:bool)  [unwired: 1 in, 1 out]
        n442 = Release Notifier(notifier=w918, force destroy? (F)=TRUE) -> ()  [unwired: 1 in, 3 out]
        n443 = property class="Bool"(reference=w923) -> ("Label.Text"=w922:string)  [unwired: 1 in, 2 out]
        n444 = call "SLM AE.vi"("Action"=enum16{"READ", "WRITE"}."READ") -> ("SLM Ref Out"=w916:refnum<vi>)  [unwired: 10 in]
        n445 = call "DM_Ref_AE.vi"("Action"=enum16{"READ", "WRITE"}."READ") -> ("DM Ref Out"=w914:refnum<vi>)  [unwired: 10 in]
        n446 = call "GateDelay AE.vi"("Action"=enum16{"READ", "WRITE"}."READ") -> ("Gate Delay Ref Out"=w915:refnum<vi>)  [unwired: 10 in]
        n447 = Enqueue Element(queue=w924, element=w922) -> ()  [unwired: 2 in, 3 out]
        n448 = Build Array(w916, w914, w915) -> (w913:refnum<vi>[])
        n449 = call "Stage_position_ae.vi"("StageID"="N664", "Enum"=enum16{"WRITE", "READ", "HOME", "SAVE HOME"}."HOME") -> ("Position Out"=w905:dbl[])  [unwired: 8 in, 1 out]
        n450 = call "Stage_position_ae.vi"("StageID"="P541", "Enum"=enum16{"WRITE", "READ", "HOME", "SAVE HOME"}."HOME") -> ("Position Out"=w909:dbl[])  [unwired: 8 in, 1 out]
        n451 = for {
          tunnel: w913 -> [w930] mode=indexing
          n452 = Not A Number/Path/Refnum?(number/path/refnum=w930) -> (NaN/Path/Refnum?=w929:bool)
          n453 = case shown="False" w929 {
            tunnel: w930 -> [w931 _]
            frame False {
              n454 = To Variant(anything=TRUE) -> (Variant=w932:variant)
              n455 = invoke class="VI" method="Ctrl Val.Set"(reference=w931, "Control Name"="Exit", "Value"=w932) -> (reference out=w935:refnum<vi>)  [unwired: 2 in, 4 out]
              n456 = Close Reference(reference=w935) -> ()  [unwired: 1 in, 1 out]
            }
            frame True {
            }
          }
        }
        n457 = Index Array(array=w905, index=0) -> (element=w902:dbl)
        n458 = property on="Stages" class="Clust (strict)"() -> ("Controls[]"=w912:refnum<vi>[])  [unwired: 2 in, 2 out]
        n459 = Index Array(array=w909, index=0) -> (element=w903:dbl)
        n460 = Build Array(w903, w902) -> (w901:dbl[])
        n461 = for {
          tunnel: w912 -> [w928] mode=indexing
          n462 = property class="Ctl"(reference=w928) -> ("Label.Text"=w927:string)  [unwired: 1 in, 2 out]
          n463 = call "All_Stages_Aloha.vi"("Aloha"=FALSE, "Stage ID"=w927) -> ()  [unwired: 9 in, 1 out]
        }
        n464 = call-poly <vilib>:"Write To Spreadsheet File.vi"("format (%.3f)"="%.4f", "1D data"=w901, "file path (dialog if empty)"=path "C:/Users/ED STED/Documents/Test Control Software/Host VIs/Stages/Stage Positions/home position.csv") -> ()  [unwired: 5 in, 1 out]
      }
    }
  }
  n465 = disable-structure shown="Disabled" {
    frame Disabled {
    }
    frame Enabled {
    }
  }
  n466 = call "Manual Controls Action Engine.vi"("Action"=enum16{"Read", "Write"}."Write", "Manual Controls In"=w27) -> ("Manual Controls Out"=w29:T18)  [unwired: 13 in]
  n467 = call "FPGA-7842R-Control V1.vi"("Action"=FPGA-7842R-Reference."Initialize", "Manual Controls"=w29, "Initialize"=FALSE) -> ("Initalized"=w11:bool)  [unwired: 11 in, 1 out]
  n468 = while {
    shift-right: [w945] -> _
    shift-left: "Idle" -> [w946]
    tunnel: w18 -> [w942]
    shift-right: [w940] -> _
    shift-left: w11 -> [w941]
    stop <- w944 stop-if-true
    n469 = call "Image Aquisition Param Ctrl_AE.vi"("Action"=enum16{"READ", "WRITE"}."READ") -> ("Image Acquisition Parameters Out"=w939:T16)  [unwired: 10 in]
    n470 = call "Detectors Crl_AE.vi"("Action"=enum16{"READ", "WRITE"}."READ") -> ("Detectors Parameters Out"=w937:T14)  [unwired: 10 in]
    n471 = case shown="\"Display\"" w946 {
      selector: w946 -> [_ _ _ w978 _ _ _ _ _ _]
      tunnel: ["Exit" w955 "Idle" ("name (unnamed)") "Arange Displays" ("name (unnamed)") "Start FPGA Acquisition" ("name (unnamed)") "Display" ("name (unnamed)") "Close Images" ("name (unnamed)") "Idle" "Stop Waveforms" ("name (unnamed)") "Start Waveforms" ("name (unnamed)")] -> w945
      tunnel: [TRUE w957 w964 w986 w1002 w1026 w1067 w1100 w1105 w1111] -> w944
      tunnel: FALSE -> [_ w957 w964 w986 w1002 w1026 w1067 w1100 w1105 w1111]
      tunnel: w942 -> [_ w956 _ _ _ _ _ _ _ _]
      tunnel: w941 -> [w951 w954 w965 w984 w999 w1024 w1065 w1098 w1106 w1112]
      tunnel: [w950 w954 w965 w984 w999 w1020 w1065 w1097 w1106 w1112] -> w940
      tunnel: w939 -> [_ _ _ w977 _ w1019 _ _ _ w1109]
      tunnel: w937 -> [_ _ _ w976 _ _ _ _ _ w1107]
      frame "Exit" {
        n472 = call "Graph Ref AE.vi"("Action"=enum16{"READ", "WRITE"}."READ") -> ("Graph Ref Out"=w948:refnum<vi>[])  [unwired: 10 in]
        n473 = call "FPGA-7842R-Control V1.vi"("Action"=FPGA-7842R-Reference."Close FPGA", "Initialize"=w951) -> ("Initalized"=w950:bool)  [unwired: 12 in, 1 out]
        n474 = Close Reference(reference=w948) -> ()  [unwired: 1 in, 1 out]
      }
      frame "Idle", Default {
        n475 = Dequeue Element(queue=w956, timeout in ms (-1)=-1) -> (element=w955:string)  [unwired: 1 in, 3 out]
      }
      frame "Close Images" {
        w960 = u16 0 items=["Read", "Write"] ("Mode")
        w961 = u16 0 items=["Write", "Read"] ("Mode")
        n476 = call "File Action V1.vi"("Mode"=w960) -> ("Files Open"=w959:bool)  [unwired: 12 in, 2 out]
        n477 = call "Image_Actions_V1.vi"("Mode"=w961, "Action"="Trash Images") -> ()  [unwired: 12 in, 2 out]
        n478 = case shown="True" w959 {
          frame False {
          }
          frame True {
            w967 = u16 1 items=["Read", "Write"] ("Mode")
            n479 = call "File Action V1.vi"("Action"="Close Files", "Mode"=w967) -> ()  [unwired: 11 in, 3 out]
          }
        }
      }
      frame "Capture", "Live" {
        w982 = u16 0 items=["Write", "Read"] ("Mode")
        n480 = Cluster To Array(cluster=w976) -> (array=w974:bool[])
        n481 = Index Array(array=w974, index=4) -> (element=w971:bool)
        n482 = Boolean To (0,1)(Boolean=w974) -> (0, 1=w975:i16[])
        n483 = Add Array Elements(numeric array=w975) -> (sum=w972:i16)
        n484 = To Long Integer(number=w972) -> (32bit integer=w969:i32)
        n485 = Unbundle By Name(w977) -> ("Image Format"=w979:u16)
        n486 = Select(t=1, s=w971, f=w969) -> (s? t:f=w968:i32)
        n487 = case shown="\"Capture\"" w978 {
          tunnel: w977 -> [_ w988]
          tunnel: w968 -> [_ w987]
          frame Default {
          }
          frame "Capture" {
            w991 = u16 1 items=["Read", "Write"] ("Mode")
            n488 = call "File Action V1.vi"("Action"="Open Files", "Mode"=w991, "Image Acquisition Parameters"=w988, "File Path IN"="Save File Path", "Number of Channels"=w987) -> ("File Path OUT"=w989:path)  [unwired: 8 in, 2 out]
            n489 = local write "Save File Path"(w989) -> ()
          }
        }
        n490 = To Long Integer(number=w979) -> (32bit integer=w981:i32)
        n491 = Bundle(w981, w981) -> (w980:cluster{i32, i32})  [unwired: 1 in]
        n492 = call "Image_Actions_V1.vi"("Image Size (Pixels)"=w980, "Mode"=w982, "Number of Channels"=w968, "Action"="Create Images") -> ()  [unwired: 10 in, 2 out]
      }
      frame "Arange Displays" {
        w997 = u16 1 items=["Write", "Read"] ("Mode")
        w1000 = u16 1 items=["Read", "Write"] ("Action")
        n493 = call "Graph Ref AE.vi"("Action"=enum16{"READ", "WRITE"}."READ") -> ("Graph Ref Out"=w993:refnum<vi>[])  [unwired: 10 in]
        n494 = call "Image_Actions_V1.vi"("Mode"=w997) -> ("Image REFs OUT"=w998:T36[])  [unwired: 13 in, 1 out]
        n495 = Array Size(array=w998) -> (size(s)=w996:i32)
        n496 = call "Arange_Displays_V2.vi"("Display References"=w993, "Action"=w1000, "Number of Channels"=w996, "Aspect Ratio (h/w)"=1.0) -> ("Number of Channels OUT"=w994:i32)  [unwired: 11 in]
        n497 = for {
          N: w994 -> [_]
          tunnel: w993 -> [w1004] mode=indexing
          tunnel: [w1007] -> _ mode=indexing
          i -> [w1005]
          n498 = property class="IntGraph (strict)"(reference=w1004) -> ("Label.Text"=w1009:string)  [unwired: 1 in, 2 out]
          n499 = Equal To 0?(x=w1005) -> (x = 0?=w1006:bool)
          n500 = case shown="True" w1006 {
            tunnel: w1004 -> [_ w1010]
            frame False {
            }
            frame True {
              n501 = property class="IntGraph (strict)"(reference=w1010, "ZScale.Visible"=TRUE ("Z Scale.Visible"), "ZScale.Position"=T25 {"Left"=2431, "Top"=-324} ("Z Scale.Position")) -> ()  [unwired: 1 in, 2 out]
            }
          }
          n502 = To Unsigned Word Integer(number=w1005) -> (unsigned 16bit integer=w1008:u16)
          n503 = Bundle("Label.Text"=w1009, w1008) -> (w1007:cluster{"Label.Text":string, u16})  [unwired: 1 in]
        }
      }
      frame "Start Waveforms" {
        n504 = Unbundle By Name("Laser Controls 2") -> ("Laser On Time (Ticks)"=w1014:i8, "Laser Delay (Ticks)"=w1013:i8)
        n505 = call "Initialize Waveforms V4.vi"("Image Acquisition Parameters"=w1019) -> ("Waveform Data to FPGA"=w1025:T37)  [unwired: 14 in]
        n506 = Unbundle By Name(w1019) -> ("Scan Type"=w1018:enum16{"Sample Scanning", "Beam Scanning"})
        n507 = call "FPGA-7842R-Control V1.vi"("Waveform Data"=w1025, "Action"=FPGA-7842R-Reference."Start Waveforms", "Laser On Time (Ticks)"=w1014, "Image Acquisition Parameters"=w1019, "Initialize"=w1024, "Laser Delay (Ticks)"=w1013) -> ("Initalized"=w1021:bool)  [unwired: 8 in, 1 out]
        n508 = Equal?(x=w1018, y=enum16{"Sample Scanning", "Beam Scanning"}."Sample Scanning" ("Scan Type")) -> (x = y?=w1016:bool)
        n509 = case shown="False" w1016 {
          tunnel: w1021 -> [w1027 w1032]
          tunnel: [w1027 w1031] -> w1020
          frame False {
          }
          frame True {
            n510 = call "Scan Parameters Action Engine.vi"("Action"=enum16{"Read", "Write"}."Read") -> ("Scan Parameters OUT"=w1029:T17)  [unwired: 14 in]
            n511 = Unbundle By Name(w1029) -> ("Unused_Axis_I16"=w1028:i16)
            n512 = call "FPGA-7842R-Control V1.vi"("Action"=FPGA-7842R-Reference."Unused Axis I16", "Initialize"=w1032, "Unused Axis Offset (I16)"=w1028) -> ("Initalized"=w1031:bool)  [unwired: 11 in, 1 out]
          }
        }
      }
      frame "Display" {
        w1060 = u16 1 items=["Write", "Read"] ("Mode")
        n513 = call "Image_Actions_V1.vi"("Mode"=w1060) -> ("Image REFs OUT"=w1062:T36[])  [unwired: 13 in, 1 out]
        n514 = Array Size(array=w1062) -> (size(s)=w1058:i32)
        n515 = Decrement(x=w1058) -> (x-1=w1057:i32)
        n516 = for {
          N: 6 -> [_]
          tunnel: w1057 -> [w1095]
          tunnel: [w1093] -> w1061 mode=indexing
          i -> [w1094]
          n517 = Greater Or Equal?(x=w1095, y=w1094) -> (x >= y?=w1093:bool)
        }
        n518 = Obtain Notifier(name (unnamed)="Running", notification data type=FALSE) -> (notifier out=w1034:refnum<notifier>)  [unwired: 2 in, 2 out]
        n519 = Index Array(array=w1061, index #1=1 ("index"), index #2=2 ("index"), index #3=3 ("index"), index #4=4 ("index"), index #5=5 ("index")) -> (element #1=w1046:bool, element #2=w1045:bool, element #3=w1044:bool, element #4=w1043:bool, element #5=w1042:bool)
        n520 = Index Array(array=w1062, index #1=0 ("index"), index #2=1 ("index"), index #3=2 ("index"), index #4=3 ("index"), index #5=4 ("index"), index #6=5 ("index")) -> (element #1=w1041:T36, element #2=w1040:T36, element #3=w1039:T36, element #4=w1038:T36, element #5=w1037:T36, element #6=w1036:T36)
        n521 = while {
          tunnel: w1046 -> [w1082]
          tunnel: w1045 -> [w1081]
          tunnel: w1044 -> [w1077]
          tunnel: w1043 -> [w1074]
          tunnel: w1042 -> [w1073]
          tunnel: w1041 -> [w1080]
          tunnel: w1040 -> [w1079]
          tunnel: w1039 -> [w1078]
          tunnel: w1038 -> [w1076]
          tunnel: w1037 -> [w1072]
          tunnel: w1036 -> [w1075]
          tunnel: w1034 -> [w1069]
          stop <- w1070 stop-if-true
          n522 = Get Notifier Status(notifier=w1069) -> (current notification=w1070:bool)  [unwired: 1 in, 4 out]
          n523 = case shown="True" w1082 {
            tunnel: w1079 -> [_ w1092]
            frame False {
            }
            frame True {
              n524 = call "IMAQ ImageToArray"("Image"=w1092) -> ("Image Pixels (Float)"=→"Channel 2":sgl[][])  [unwired: 3 in, 4 out]
            }
          }
          n525 = case shown="True" w1081 {
            tunnel: w1078 -> [_ w1090]
            frame False {
            }
            frame True {
              n526 = call "IMAQ ImageToArray"("Image"=w1090) -> ("Image Pixels (Float)"=→"Channel 3":sgl[][])  [unwired: 3 in, 4 out]
            }
          }
          n527 = call "IMAQ ImageToArray"("Image"=w1080) -> ("Image Pixels (Float)"=→"Channel 1":sgl[][])  [unwired: 3 in, 4 out]
          n528 = case shown="True" w1077 {
            tunnel: w1076 -> [_ w1088]
            frame False {
            }
            frame True {
              n529 = call "IMAQ ImageToArray"("Image"=w1088) -> ("Image Pixels (Float)"=→"Channel 4":sgl[][])  [unwired: 3 in, 4 out]
            }
          }
          n530 = case shown="False" w1074 {
            tunnel: w1072 -> [_ w1086]
            frame False {
            }
            frame True {
              n531 = call "IMAQ ImageToArray"("Image"=w1086) -> ("Image Pixels (Float)"=→"Channel 5":sgl[][])  [unwired: 3 in, 4 out]
            }
          }
          n532 = case shown="True" w1073 {
            tunnel: w1075 -> [_ w1084]
            frame False {
            }
            frame True {
              n533 = call "IMAQ ImageToArray"("Image"=w1084) -> ("Image Pixels (Float)"=→"Channel 6":sgl[][])  [unwired: 3 in, 4 out]
            }
          }
          n534 = Wait (ms)(milliseconds to wait=u32 100) -> ()  [unwired: 1 out]
        }
      }
      frame "Stop Waveforms" {
        n535 = call "FPGA-7842R-Control V1.vi"("Action"=FPGA-7842R-Reference."Stop Waveforms", "Initialize"=w1098) -> ("Initalized"=w1097:bool)  [unwired: 12 in, 1 out]
      }
      frame "Stop Acquisition" {
        n536 = call "FPGA-7842R-Control V1.vi"("Action"=FPGA-7842R-Reference."Laser Control", "Laser Controls"=T15 {"STED Power (V)"=0.0, "STED"=FALSE, "650 nm"=FALSE, "590 nm"=FALSE, "485 nm"=FALSE, "Manual Control"=FALSE} ("Laser Controls 2"), "Initialize"=TRUE) -> ()  [unwired: 11 in, 2 out]
      }
      frame "Start FPGA Acquisition" {
        n537 = Unbundle By Name(w1109) -> ("Scan Mode"=w1108:enum16{"XY", "XZ", "YZ", "XYZ"})
        n538 = case shown="\"XZ\", Default" w1108 {
          tunnel: w1109 -> [_ w1119]
          tunnel: w1107 -> [_ w1120]
          frame "YZ" {
            n539 = vi-ref "FPGA Sample Scanning V1.vi"() -> (w1115:refnum<vi>)
            n540 = property class="VI Interface Type 3"(reference=w1115) -> ("Path"=w1113:path)  [unwired: 1 in, 2 out]
            n541 = Open VI Reference(type specifier VI Refnum (for type only)=w1115, vi path=w1113, options=128) -> (vi reference=w1116:refnum<vi>)  [unwired: 3 in, 1 out]
            n542 = call-by-ref "Start Asynchronous Call"(reference=w1116) -> (reference out=w1117:refnum<vi>)  [unwired: 4 in, 1 out]
            n543 = Close Reference(reference=w1117) -> ()  [unwired: 1 in, 1 out]
          }
          frame "XZ", Default {
            n544 = vi-ref "FPGA Beam Scanning V1.vi"() -> (w1118:refnum<vi>)
            n545 = property class="VI Interface Type 4"(reference=w1118) -> ("Path"=w1122:path)  [unwired: 1 in, 2 out]
            n546 = Open VI Reference(type specifier VI Refnum (for type only)=w1118, vi path=w1122, options=128) -> (vi reference=w1121:refnum<vi>)  [unwired: 3 in, 1 out]
            n547 = call-by-ref "Start Asynchronous Call"(reference=w1121, "Detectors"=w1120, "Image Acquisition Parameters"=w1119) -> (reference out=w1124:refnum<vi>)  [unwired: 2 in, 1 out]
            n548 = Close Reference(reference=w1124) -> ()  [unwired: 1 in, 1 out]
          }
        }
      }
    }
  }
